vi "Dashboard Main.vi"() -> ()   [LabVIEW 2023]
uses:
  <vilib>/Utility/miscctls.llb/LVRectTypeDef.ctl
  <vilib>/event_ctls.llb/eventvkey.ctl
  <vilib>/Rock Robotics/WPI/DriverStation/WPI_DriverStationAllianceInfo.ctl
  <vilib>/robotics/Kinematics/DH Kinematic Parameters.ctl
  <vilib>/robotics/Kinematics/Link/Joint Type.ctl
  b1c29fd4-b69e-4c47-bd92-218700034153.vi
  cd51690b-7cbe-44fb-a5f0-3232adb0ed53.vi
  a4e8d5d1-2ec3-4e81-be0b-60391cc68073.vi
  1b78be80-bab2-445d-a3e8-82f142a16380.vi
  9e807339-2903-4f51-8fcc-64b6a9381567.vi
  e75f20ac-3dfa-4544-8614-4803d6d17fbb.vi
  273c17a0-a238-4f2a-a55a-7e29d73850ff.vi
  87bdd142-1820-4e26-8582-f713a5f3da40.vi
  b8451b18-7b16-4e07-a196-a1bebf8ce026.vi
  5d307e9f-edd0-4132-a387-09c5916d43b1.vi
  0137daef-9682-45ba-80b9-2d4fda8852b8.vi
  f6a63fab-964b-4051-8314-d4414a0a258c.vi
  90e0fe9d-42b1-4a72-a6c8-4b9d9b3a5a2a.vi
  f15e925d-3118-43e3-bf67-a1272bbf81dd.vi
  394886aa-4cdd-4740-8681-89e3e438764a.vi
  77a42c1f-99bf-4bb6-8218-45b49017f7dc.vi
  5abae45b-ab2b-4816-ba0c-2a0b218f6531.vi
  31f70c1d-3051-4c77-9544-a691198ba614.vi
  f63f5451-5db6-487e-bc86-5cb81e92b132.vi
  81d0db6a-d68a-45c3-b3b1-458879412541.vi
  c235c188-eb56-46fb-93d3-e8acf396af31.vi
  115ba94a-0b26-47fa-ae73-5ec5bd9e502a.vi
  2422668c-951b-48e5-9bda-0f59c56d9c0d.vi
  7776664e-4af7-4b3d-b288-2266642a045e.vi
  321ce103-7778-4bb1-9ecc-75a76fef05e9.vi
  d30e88cc-5e2b-4867-b271-53fc6d5cd4d7.vi
  fde90579-e212-4b8a-8145-a17c3e40bcbd.vi
  6c63589b-432e-4f9c-bacb-2063ed7bd576.vi
  b7dcf304-99f6-4f78-9d14-19aa8d9ea562.vi
  e8b3bb93-ba91-445b-94c6-9e998421f827.vi
  0480a820-69ef-45e6-a9f4-d7ff60c89e45.vi
  1c99237e-ea3d-4ecf-b7c2-61034db3ecd2.vi
  7f172f69-595e-4449-a51b-8be7e20a4729.vi
  02f5d99f-024f-4135-b77d-0032ba8d795b.vi
  0004bdb2-d360-448a-aeac-771fcc1baf3b.vi
  92b8c23e-1d1c-4057-b5e6-223c27eaed30.vi
  7dffb039-adaa-4868-8e10-c58d0581d4f2.vi
  0eb6f919-4c91-4ba7-8f64-447c9ee320a2.vi
  51c227ae-7212-4b29-a489-1f89dd7475d1.vi
  ccddf429-f836-4a79-b987-12239753ca83.vi
  ce254ba4-3e57-42c7-9282-1ab8c635dc3e.vi
  29e0c3c6-4e3c-47cb-b565-5e4554484683.vi
  0a8fe2ab-d060-4915-a9b5-d8978247e2b6.vi
  b1c29fd4-b69e-4c47-bd92-218700034153.vi/77c742ae-e671-49bb-a825-a6e8cebc9f63.vi
  cd51690b-7cbe-44fb-a5f0-3232adb0ed53.vi/77c742ae-e671-49bb-a825-a6e8cebc9f63.vi
  a4e8d5d1-2ec3-4e81-be0b-60391cc68073.vi/77c742ae-e671-49bb-a825-a6e8cebc9f63.vi
  1b78be80-bab2-445d-a3e8-82f142a16380.vi/77c742ae-e671-49bb-a825-a6e8cebc9f63.vi
  9e807339-2903-4f51-8fcc-64b6a9381567.vi/77c742ae-e671-49bb-a825-a6e8cebc9f63.vi
  e75f20ac-3dfa-4544-8614-4803d6d17fbb.vi/77c742ae-e671-49bb-a825-a6e8cebc9f63.vi
  0137daef-9682-45ba-80b9-2d4fda8852b8.vi/77c742ae-e671-49bb-a825-a6e8cebc9f63.vi
  f6a63fab-964b-4051-8314-d4414a0a258c.vi/77c742ae-e671-49bb-a825-a6e8cebc9f63.vi
  90e0fe9d-42b1-4a72-a6c8-4b9d9b3a5a2a.vi/77c742ae-e671-49bb-a825-a6e8cebc9f63.vi
  f15e925d-3118-43e3-bf67-a1272bbf81dd.vi/77c742ae-e671-49bb-a825-a6e8cebc9f63.vi
  394886aa-4cdd-4740-8681-89e3e438764a.vi/77c742ae-e671-49bb-a825-a6e8cebc9f63.vi
  77a42c1f-99bf-4bb6-8218-45b49017f7dc.vi/77c742ae-e671-49bb-a825-a6e8cebc9f63.vi
  5abae45b-ab2b-4816-ba0c-2a0b218f6531.vi/77c742ae-e671-49bb-a825-a6e8cebc9f63.vi
  31f70c1d-3051-4c77-9544-a691198ba614.vi/77c742ae-e671-49bb-a825-a6e8cebc9f63.vi
  f63f5451-5db6-487e-bc86-5cb81e92b132.vi/77c742ae-e671-49bb-a825-a6e8cebc9f63.vi
  81d0db6a-d68a-45c3-b3b1-458879412541.vi/77c742ae-e671-49bb-a825-a6e8cebc9f63.vi
  c235c188-eb56-46fb-93d3-e8acf396af31.vi/77c742ae-e671-49bb-a825-a6e8cebc9f63.vi
  115ba94a-0b26-47fa-ae73-5ec5bd9e502a.vi/77c742ae-e671-49bb-a825-a6e8cebc9f63.vi
  2422668c-951b-48e5-9bda-0f59c56d9c0d.vi/77c742ae-e671-49bb-a825-a6e8cebc9f63.vi
  7776664e-4af7-4b3d-b288-2266642a045e.vi/77c742ae-e671-49bb-a825-a6e8cebc9f63.vi
  321ce103-7778-4bb1-9ecc-75a76fef05e9.vi/77c742ae-e671-49bb-a825-a6e8cebc9f63.vi
  d30e88cc-5e2b-4867-b271-53fc6d5cd4d7.vi/77c742ae-e671-49bb-a825-a6e8cebc9f63.vi
  fde90579-e212-4b8a-8145-a17c3e40bcbd.vi/77c742ae-e671-49bb-a825-a6e8cebc9f63.vi
  6c63589b-432e-4f9c-bacb-2063ed7bd576.vi/77c742ae-e671-49bb-a825-a6e8cebc9f63.vi
  b7dcf304-99f6-4f78-9d14-19aa8d9ea562.vi/77c742ae-e671-49bb-a825-a6e8cebc9f63.vi
  e8b3bb93-ba91-445b-94c6-9e998421f827.vi/77c742ae-e671-49bb-a825-a6e8cebc9f63.vi
  0480a820-69ef-45e6-a9f4-d7ff60c89e45.vi/77c742ae-e671-49bb-a825-a6e8cebc9f63.vi
  1c99237e-ea3d-4ecf-b7c2-61034db3ecd2.vi/77c742ae-e671-49bb-a825-a6e8cebc9f63.vi
  <vilib>/robotics/Kinematics/RotateX.vi
  <vilib>/robotics/Kinematics/RotateY.vi
  <vilib>/robotics/Kinematics/RotateZ.vi
  <vilib>/Analysis/baseanly.llb/A x B.vi
  <vilib>/Analysis/baseanly.llb/Real A x B.vi
  7f172f69-595e-4449-a51b-8be7e20a4729.vi/77c742ae-e671-49bb-a825-a6e8cebc9f63.vi
  02f5d99f-024f-4135-b77d-0032ba8d795b.vi/77c742ae-e671-49bb-a825-a6e8cebc9f63.vi
  0004bdb2-d360-448a-aeac-771fcc1baf3b.vi/77c742ae-e671-49bb-a825-a6e8cebc9f63.vi
  92b8c23e-1d1c-4057-b5e6-223c27eaed30.vi/77c742ae-e671-49bb-a825-a6e8cebc9f63.vi
  7dffb039-adaa-4868-8e10-c58d0581d4f2.vi/77c742ae-e671-49bb-a825-a6e8cebc9f63.vi
  29e0c3c6-4e3c-47cb-b565-5e4554484683.vi/77c742ae-e671-49bb-a825-a6e8cebc9f63.vi
  0a8fe2ab-d060-4915-a9b5-d8978247e2b6.vi/77c742ae-e671-49bb-a825-a6e8cebc9f63.vi
  <vilib>/Rock Robotics/Network Tables/NT Read Number.vi
  <vilib>/Rock Robotics/Network Tables/NT Read Boolean.vi
  GlobalDashboard.vi
  <vilib>/Rock Robotics/Network Tables/NT Read String.vi
  <vilib>/Rock Robotics/Network Tables/NT Write Number.vi
  <vilib>/Rock Robotics/Network Tables/NT Read Numeric Array.vi
  <vilib>/Rock Robotics/Network Tables/NT Read String Array.vi
  <vilib>/Rock Robotics/Network Tables/NT Write Boolean.vi
  <vilib>/Rock Robotics/Network Tables/NT Read Boolean Array.vi
  <vilib>/Rock Robotics/Network Tables/NT Write String.vi
  <vilib>/Rock Robotics/Network Tables/NT Write Numeric Array.vi
  <vilib>/picture/3D Picture Control/Object/Add Object (no reference).vi
  <vilib>/Rock Robotics/Network Tables/NT Write String Array.vi
  <vilib>/Utility/xml.llb/Write to XML File(string).vi
  <vilib>/Utility/xml.llb/Read From XML File(array).vi
  <vilib>/picture/3D Picture Control/Object/Create Object (drawable).vi
  <vilib>/Rock Robotics/Network Tables/NT Read Integer.vi
  <vilib>/robotics/Kinematics/Analytical/Initialize Generic Serial Arm.vi
  <vilib>/vision/NI_Vision_Development_Module.lvlib
  <vilib>/robotics/Kinematics/Link/NI_Robotics_Link.lvclass
  <vilib>/robotics/Kinematics/Analytical/NI_Robotics_AnalyticKinematics.lvlib
  <vilib>/robotics/Kinematics/Robot/NI_Robotics_Serial Robot Arm.lvclass
  <vilib>/robotics/Kinematics/NI_Kinematics.lvlib
  <vilib>/picture/3D Picture Control/NI_3D Picture Control.lvlib
  <vilib>/robotics/Kinematics/Plotting/NI_Robotics_3DKinematics.lvlib
panel:
  out "Shooter_Fault_Array":bool[](array[boolean])
  out "Shooter_Overheating_Array":bool[](array[boolean])
  in  "TCP":refnum<k5>
  in  "Dashboard Tab":T1(tab)=enum."Setup/Auto"
  in  "CheckList":i32(listbox)
  in  "Launch_Camera":bool
  out "Distance_to_Target":dbl format="%.1f"
  in  "Enable_Streaming_GUI":bool=TRUE
  out "Robot_Profile_GUI":string
  out "Auto_Playbook_GUI":string
  in  "Select Driver Profile":u16(ring) items=["N/A"]
  in  "Camera Name":string(combo)="limelight"
  in  "Camera Settings":T2={"Frame Rate"=20, "Compression"=60, "Size"=1, "DB Camera Config"=FALSE} {"Size" items=["640x480", "320x240", "160x120"]}
  in  "Select Autonomous Play":u16(ring) items=["N/A"]
  out "Master_Caution_GUI_0":bool caption="Mode_Butterfly"
  out "Robot_is_Autonomous_GUI_0":bool caption="Mode_Butterfly"
  out "Robot_Code_Version_GUI":string
  out "Auto_Suffix_GUI":string
  in  "Refresh_Auto_Play_List_GUI":bool
  in  "Auto_Delay_GUI":dbl format="%.1f"
  in  "Manual_Start_X":dbl min=0.0 max=700.0 format="%.1f"
  out "Robot_X":dbl format="%.1f"
  out "Robot_Y":dbl format="%.1f"
  in  "Manual_Start_Y":dbl min=0.0 max=400.0 format="%.1f"
  out "Robot_H_GUI":dbl format="%.1f"
  in  "Manual_Start_H":dbl min=0.0 max=360.0 format="%.1f"
  in  "Field Map":u16(ring) items=["N/A"]
  in  "Push_Robot_Start_GUI":bool
  in  "Export_Robot_Pose":bool
  in  "Clear_Robot_Pose_Display":bool
  in  "Dock_Dashboard":bool
  in  "Force_Human_Control_GUI":bool
  in  "Auto_Test_Mode_GUI":bool
  in  "Disable_Fusion_While_Autonomous":bool
  in  "Disable_Fusion_While_Disabled":bool=TRUE
  out "Robot Pose 1":cluster{dbl[], dbl[]}[](graph)
  in  "Camera Switch\nCamera Switch":bool
  out "Master_State_STOW_Indicator":bool
  in  "Elevator_Override":bool
  in  "Wrist_Override":bool
  out "(Front) Lemon_Vision_Fault_GUI":bool
  out "Shooter_State_STGE":bool
  out "Shooter_State_SUBW":bool
  out "Shooter_State_TACO":bool
  out "Note 2":bool caption="Mode_Butterfly"
  out "Wrist_Motor_Fault":bool
  out "Wrist_Overheating":bool
  out "Ready_To_Fire":bool caption="Mode_Butterfly"
  out "Shooter_Right_Overheating":bool
  out "Shooter_Motor_Right_Fault":bool
  out "Outtaking":bool caption="Mode_Butterfly"
  out "Intaking":bool caption="Mode_Butterfly"
  out "Shooter_Motor_Left_Fault":bool
  out "Shooter_Left_Overheating":bool
  out "Indexer_Overheating":bool
  out "Indexer_Motor_Fault":bool
  out "Intake_Motor_Fault":bool
  out "Intake_Overheating":bool
  out "Elevator_Motor_Fault":bool
  out "Elevator_Overheating":bool
  out "Master_State_TRAP_Indicator":bool
  out "Master_State_CLIMB_Indicator":bool
  out "Master_State_AMP_Indicator":bool
  out "Help Graphic":T3(plugin-control)
  out "LL_Ret_Left":bool
  out "LL_Ret_Right":bool
  out "WA_Ret_Right":bool
  out "WA_Ret_Left":bool
  out "Swerve_Drive_Fault":bool
  out "Robot Pose 2":cluster{dbl[], dbl[]}[](graph)
  out "Master_State_SPEAKER_Indicator":bool
  out "(Back) Lime_Vision_Fault_GUI":bool
  out "Pressure_Leak_GUI":bool
  in  "Master_Safety_Override_1":bool
  in  "Manipulator_Help":bool
  in  "Driver_Help":bool
  out "No_Secondary_Camera":bool
  out "Electrical_Fault_GUI":bool
  out "Diverting_Power_GUI":bool
  out "CAN_Bus_Fault_GUI":bool
  out "IMU_Failure_GUI":bool
  out "Robot_is_Autonomous_GUI_1":bool caption="Mode_Butterfly"
  out "LL_Valid":bool caption="Mode_Butterfly"
  out "Auto_Error_GUI":bool
  in  "Clear_Errors_GUI":bool
  out "Swerve_Azimuth_Fault":bool
  out "Pressure_Transducer_GUI":dbl(slide) scale=0.0..115.0
  out "Pressure_Vent_GUI":bool
  out "Swerve_Overheating":bool
  out "Compressor_On_GUI":bool
  in  "Right":bool
  in  "Reticule":T4(ring)
  in  "Save":bool
  in  "Up":bool
  in  "Down":bool
  in  "Left":bool
  out "Master_Caution_GUI_1":bool caption="Mode_Butterfly"
  out "Battery_Critical_GUI":bool
  out "Battery_Voltage_GUI":dbl(slide) scale=11.0..13.0
  out "Field_Oriented_GUI":bool caption="Mode_Butterfly"
  out "Slow_Loop":bool
  out "Combined Camera Feed":T3(plugin-control)
  in  "Field_Oriented_Override_GUI":bool
  in  "Auto_Targeting_Override":bool
  out "Using_Auto_Targeting":bool caption="Mode_Butterfly"
  out "Elevator_Has_Arrived":bool caption="Mode_Butterfly"
  out "Pivot_Position (deg)":dbl format="%.1f"
  out "Pivot_Temp (C)":dbl
  in  "Unlock_Pivot":bool
  out "Wrist_Position (deg) 2":dbl format="%.1f"
  out "Wrist_Temp (C) 2":dbl
  in  "Unlock_Wrist":bool
  out "Swerve_Output_Loop_Time_GU":u32
  out "Swerve_3_Drive_Velocity":dbl format="%.1f"
  out "Swerve_3_Azimuth_Position":dbl format="%.1f"
  out "Swerve_3_Drive_Temperature":dbl
  out "Swerve_0_Drive_Temperature":dbl
  out "Camera Perf":string
  out "Control_Loop_Time_GUI":u32
  in  "Calibrate_Wheels_GUI":bool
  in  "Home_Wheels_GUI":bool
  out "Swerve_0_Azimuth_Position":dbl format="%.1f"
  out "Swerve_0_Drive_Velocity":dbl format="%.1f"
  out "Swerve_1_Drive_Velocity":dbl format="%.1f"
  out "Swerve_1_Azimuth_Position":dbl format="%.1f"
  out "Swerve_1_Drive_Temperature":dbl
  out "Swerve_2_Drive_Velocity":dbl format="%.1f"
  out "Swerve_2_Azimuth_Position":dbl format="%.1f"
  out "Swerve_2_Drive_Temperature":dbl
  in  "Arm_Calibrate_Wheels_GUI":bool
  out "Master_Caution_GUI_2":bool caption="Mode_Butterfly"
  in  "Actuator Testing":u16(ring) items=["N/A"]
  in  "Test_Actuator_Value_GUI":dbl step=0.1 format="%.2f"
  in  "Calibrate_Joysticks_GUI":bool
  in  "Arm_Calibrate_Joysticks":bool
  out "Robot_is_Autonomous_GUI_2":bool caption="Mode_Butterfly"
  in  "Test_Actuator_Period_GUI":dbl min=0.0 step=1.0 format="%.2f"
  out "Pose_Loop_Time_GUI":u32
  in  "Mute_Audible_Warnings":bool
  out "Combined Error String":string
  out "Swerve_0_Shifter_State":string
  out "Swerve_1_Shifter_State":string
  out "Swerve_3_Shifter_State":string
  out "Swerve_2_Shifter_State":string
  out "Swerve_Azimuth_Fault_Array":bool[](array[boolean])
  in  "Super_Test_Mode_GUI":bool
  out "Current_Driver_Profile_Setpoints_GUI":T5={"Strafe Deadband"=0.08, "Strafe Scaling"=2.0, "Strafe Maximum"=0.5, "Rotation Deadband"=0.15, "Rotation Scaling"=2.5, "Rotation Maximum"=0.5} {"Rotation Maximum" min=0.3 max=1.0 scale=0.3..1.0; "Rotation Scaling" min=1.0 max=4.0 scale=1.0..4.0; "Rotation Deadband" min=0.0 max=0.25 scale=0.0..0.25; "Strafe Maximum" min=0.3 max=1.0 scale=0.3..1.0; "Strafe Scaling" min=1.0 max=4.0 scale=1.0..4.0; "Strafe Deadband" min=0.0 max=0.25 scale=0.0..0.25}
  in  "New_Driver_Profile_Setpoints_GUI":T6={"Strafe Deadband"=0.08, "Strafe Scaling"=2.0, "Strafe Max"=0.5, "Rotate Deadband"=0.15, "Rotate Scaling"=2.5, "Rotate Max"=0.5} {"Rotate Max" min=0.3 max=1.0 format="%.2g"; "Rotate Scaling" min=1.0 max=4.0 format="%.2g"; "Rotate Deadband" min=0.0 max=0.25 format="%.2g"; "Strafe Max" min=0.3 max=1.0 format="%.2g"; "Strafe Scaling" min=1.0 max=4.0 format="%.2g"; "Strafe Deadband" min=0.0 max=0.25 format="%.2g"}
  in  "Apply_Driver_Profile_Setpoints_GUI":bool
  out "Current_Driver_Profile_GUI":string
  in  "Free_Tuning_Variable_GUI":dbl min=0.0 step=1.0 format="%.3f"
  out "Audible_Warnings_Enabled_GUI":bool
  out "Legal_Drivers_GUI":string[](array[string])
  out "Swerve_Overheating_Array":bool[](array[boolean])
  out "Swerve_Drive_Fault_Array":bool[](array[boolean])
  out "Intake_Motor_Fault_Array":bool[](array[boolean])
  out "Intake_Overheating_Array":bool[](array[boolean])
  out "Extender_Position (deg)":dbl format="%.1f"
  out "Extender_Temp (C)":dbl
  in  "Calibrate_Extender":bool
  in  "Unlock_Extender":bool
  out "State_AMP":bool
  out "State_Climbing":bool
  out "NT Connection":bool
  out "Mode":T7(ring)=enum."Auto Disabled"
  out "Tree":string(tree)
  out "Background":bool
  # "2025 Dashboard v1.0-dev"
  # "Robot Profile"
  # "Robot X Position (in)"
  # "Robot Y Position (in)"
  # "Delay (s)"
  # "Robot Heading (deg)"
  # "Suffix"
  # "X (in)"
  # "Robot Pitch (deg)"
  # "Autonomous Playbook Entry"
  # "Auto Test\nMode"
  # "Force\nHuman"
  # "Y (in)"
  # "Target Distance (in)"
  # "H (deg)"
  # "Undock Dashboard"
  # "Yes Camera Streaming"
  # "Stop Fusion While Auto"
  # "Stop Fusion While Disabled"
  # "X"
  # "Y"
  # "MASTER\nSTATES"
  # "OVERRIDES"
  # "Robot-Oriented Drive Controls"
  # "Camera Switch"
  # "Auto-Targeting Override"
  # "Wrist\nOverride"
  # "SHOOTER\nSTATES"
  # "Arm\nOverride"
  # "Disengage\nSafeties"
  # "11"
  # "13"
  # "0"
  # "120"
  # "Drivebase Subsytem"
  # "Driver Profile Selected"
  # "Loop Times"
  # "Module 1"
  # "Module 0"
  # "Control (ms)"
  # "Azimuth (deg)"
  # "Pose (ms)"
  # "Temp (C)"
  # "Drive Output (ms)"
  # "Velocity (ft/s)"
  # "Shifter State"
  # "Module 2"
  # "Module 3"
  # "Variable (bleh)"
  # "Disabled\nTest Mode"
  # "Azimuth (deg)"
  # "Temp (C)"
  # "Velocity (ft/s)"
  # "Arm Subsystem"
  # "Shifter State"
  # "Calibrate Extender"
  # "Unlock Wrist"
  # "Unlock Pivot"
  # "Calibrate Wheels"
  # "Gripper Subsystem"
  # "Extender"
  # "Extender"
  # "Extender"
  # "Period (s)"
  # "Calibrate Joysticks"
  # "Amplitude"
  # "Velocity (rpm)"
  # "Position (in)"
  # "Pos (deg)"
  # "Pos (deg)"
  # "Temp (C)"
  # "Temp (C)"
  # "Temp (C)"
  # "Temp (C)"
  # "0"
  # "0.25"
  # "1"
  # "4"
  # "0.3"
  # "1"
  # "0"
  # "0.25"
  # "1"
  # "4"
  # "0.3"
  # "1"
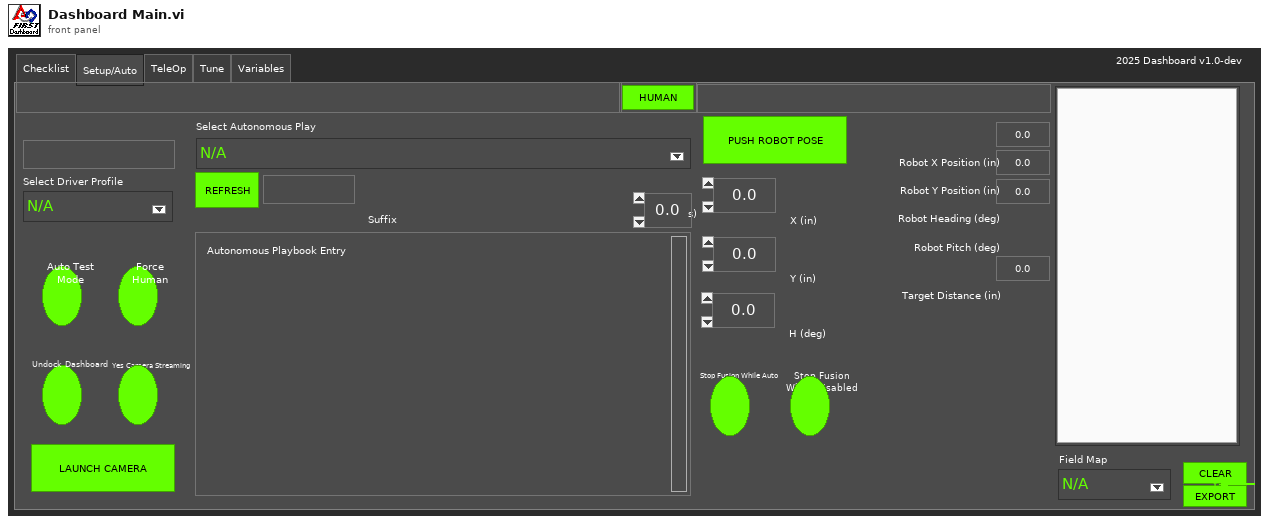
[diagram p1: front panel]
types:
  T1 = enum32{"Checklist", "Setup/Auto", "TeleOp", "Tune", "NT", "Test", "Commands", "Variables"}
  T2 = cluster{"Frame Rate":i32, "Compression":i32, "Size":u16, "DB Camera Config":bool}
  T3 = typedef "IMAQ Image.ctl" = refnum<image>
  T4 = enum16{"Wide Angle Left Reticule", "Wide Angle Right Reticule", "Lime Light Left Reticule", "Lime Light Right Reticule"}
  T5 = cluster{"Strafe Deadband":dbl, "Strafe Scaling":dbl, "Strafe Maximum":dbl, "Rotation Deadband":dbl, "Rotation Scaling":dbl, "Rotation Maximum":dbl}
  T6 = cluster{"Strafe Deadband":dbl, "Strafe Scaling":dbl, "Strafe Max":dbl, "Rotate Deadband":dbl, "Rotate Scaling":dbl, "Rotate Max":dbl}
  T7 = enum8{"Tele-Op Disabled", "Tele-Op Enabled", "Auto Disabled", "Auto Enabled", "Test Disabled", "Test Enabled", "Disconnected", "No Code", "E-Stop"}
  T8 = cluster{"Save Path":path, "Interval (s)":dbl, "Keep":i32}
  T9 = enum32{"Drive", "Camera", "Basic", "Custom", "Test", "Commands", "Checklist", "Variables"}
  T10 = cluster{"IDs":cluster{"RPC field ID":u16, "Unique ID":u16}, "String":string}
  T11 = typedef "Image Type" = u32
  T12 = cluster{"Camera Name":string, string, "Saved DB Images Info":cluster{"Save Path":path, "Interval (s)":dbl, "Keep":i32}}
  T13 = typedef "WPI_DriverStationAllianceInfo.ctl" = enum16{"Red", "Blue", "Invalid"}
  T14 = cluster{"Red":sgl, "Green":sgl, "Blue":sgl, "Alpha":sgl}
  T15 = typedef "DH Kinematic Parameters.ctl" = cluster{"twist angle":dbl, "length":dbl, "rotation angle":dbl, "offset distance":dbl, "joint type":T16, "joint coordinate offset":dbl}
  T16 = typedef "NI_Robotics_Link.lvclass/Joint Type.ctl" = enum16{"Revolute", "Prismatic"}
  T17 = enum8{"Enabled", "Disabled", "Disabled and Grayed Out"}
  T18 = cluster{"Error Strings":string, "Disable Counts":cluster{u16, u16}, "Rail Faults":cluster{u16, u16, u16}, "Robot IP":string, "DB Mode":u8, "Event Info":cluster{"Name":string, "Type":u8, "Number":u16, "Replay":u8}}
  T19 = cluster{"Storage":cluster{"Disk Free":u64, "RAM Block":u32, "RAM free":u32}, "CPU Utilization":cluster{"CPU % ISR":sgl, "CPU % Time Crit":sgl, "CPU % Timed Str":sgl, "CPU % High":sgl, "CPU % Above":sgl, "CPU % Normal":sgl, "CPU % Low":sgl}, "CAN":cluster{"% Bus Utilization":sgl, "Bus Off Cnt":u32, "TX_FIFO Full Cnt":u32, "Receive Error Cnt":u8, "Transmit Error Cnt":u8}, "HID":cluster{"HID Outputs":u32, "Rumble Low":u16, "Rumble High":u16}[]}
  T20 = cluster{"Status bits":cluster{"Test Mode":bool, "Autonomous":bool, "Enabled":bool, "Code Start":bool, "Brownout":bool, "Reserved 2":bool, "Reserved 3":bool, "E-Stop":bool}, "Code Trace":cluster{"Disabled":bool, "TeleOp":bool, "Auto":bool, "Test":bool}, "Controller Type":enum16{"unknown", "cRIO", "roboRio"}, "Code?":enum16{"unknown", "noCode", "code"}, "Battery V":dbl}
  T21 = cluster{"Control Bits":cluster{"TestMode":bool, "Autonomous":bool, "Enabled":bool, "FMS Present":bool, bool, bool, bool, "E-Stop":bool}, "Team Station ":u8, "Countdown":sgl, "Joystick Values":cluster{"Axes":dbl[], "Buttons":bool[], "POVs":i16[]}[]}
  T22 = typedef "imagedata.ctl" = cluster{"image type":i32, "image depth":i32, "image":u8[], "mask":u8[], "colors":u32[], "Rectangle":cluster{"left":i16, "top":i16, "right":i16, "bottom":i16}}
  T23 = cluster{"Boolean":bool, "Numeric Text.Text Colors:Text Color":u32}
  T24 = cluster{"value[0]":dbl, "value[1]":dbl, "value[2]":dbl, "value[3]":dbl, "value[4]":dbl, "value[5]":dbl}
  T25 = typedef "NI_Matrix.lvlib/RealMatrix.ctl" = dbl[][]
  T26 = typedef "LVRectTypeDef.ctl" = cluster{"Left":i16, "Top":i16, "Right":i16, "Bottom":i16}
  T27 = typedef "eventvkey.ctl" = enum16{"ASCII", "Enter", "Return", "Shift", "Ctrl", "Alt", "Cmd", "Opt", "Caps", "NumLock", "Clear", "Break", "Up", "Down", "Left", "Right", "Insert", "Delete", "Home", "End", "PageUp", "PageDown", "Escape", "Help", "Pause", "ScrollLock", "F1", "F2", "F3", "F4", "F5", "F6", "F7", "F8", "F9", "F10", "F11", "F12", "F13", "F14", "F15", "F16", "F17", "F18", "F19", "F20", "F21", "F22", "F23", "F24", "Play", "VolumeUp", "VolumeDown", "Mute", "Two Byte Char"}
  T28 = cluster{"Shift":bool, "Ctrl":bool, "Alt":bool, "Cmd":bool, "Opt":bool}
  T29 = cluster{"WA_Ret_Left":refnum<vi>, "WA_Ret_Right":refnum<vi>, "LL_Ret_Left":refnum<vi>, "LL_Ret_Right":refnum<vi>}
  T30 = cluster{string, "(Back) Lime_Vision_Fault_GUI":bool, dbl}
  T31 = cluster{string, "Elevator_Motor_Fault":bool, dbl}
  T32 = cluster{string, "Elevator_Overheating":bool, dbl}
  T33 = cluster{string, "Master_Safety_Override_1":bool, dbl}
  T34 = cluster{string, "Swerve_Azimuth_Fault":bool, dbl}
  T35 = cluster{string, "Arm_Calibrate_Wheels_GUI":bool, dbl}
  T36 = cluster{string, "Electrical_Fault_GUI":bool, dbl}
  T37 = cluster{string, "Arm_Calibrate_Joysticks":bool, dbl}
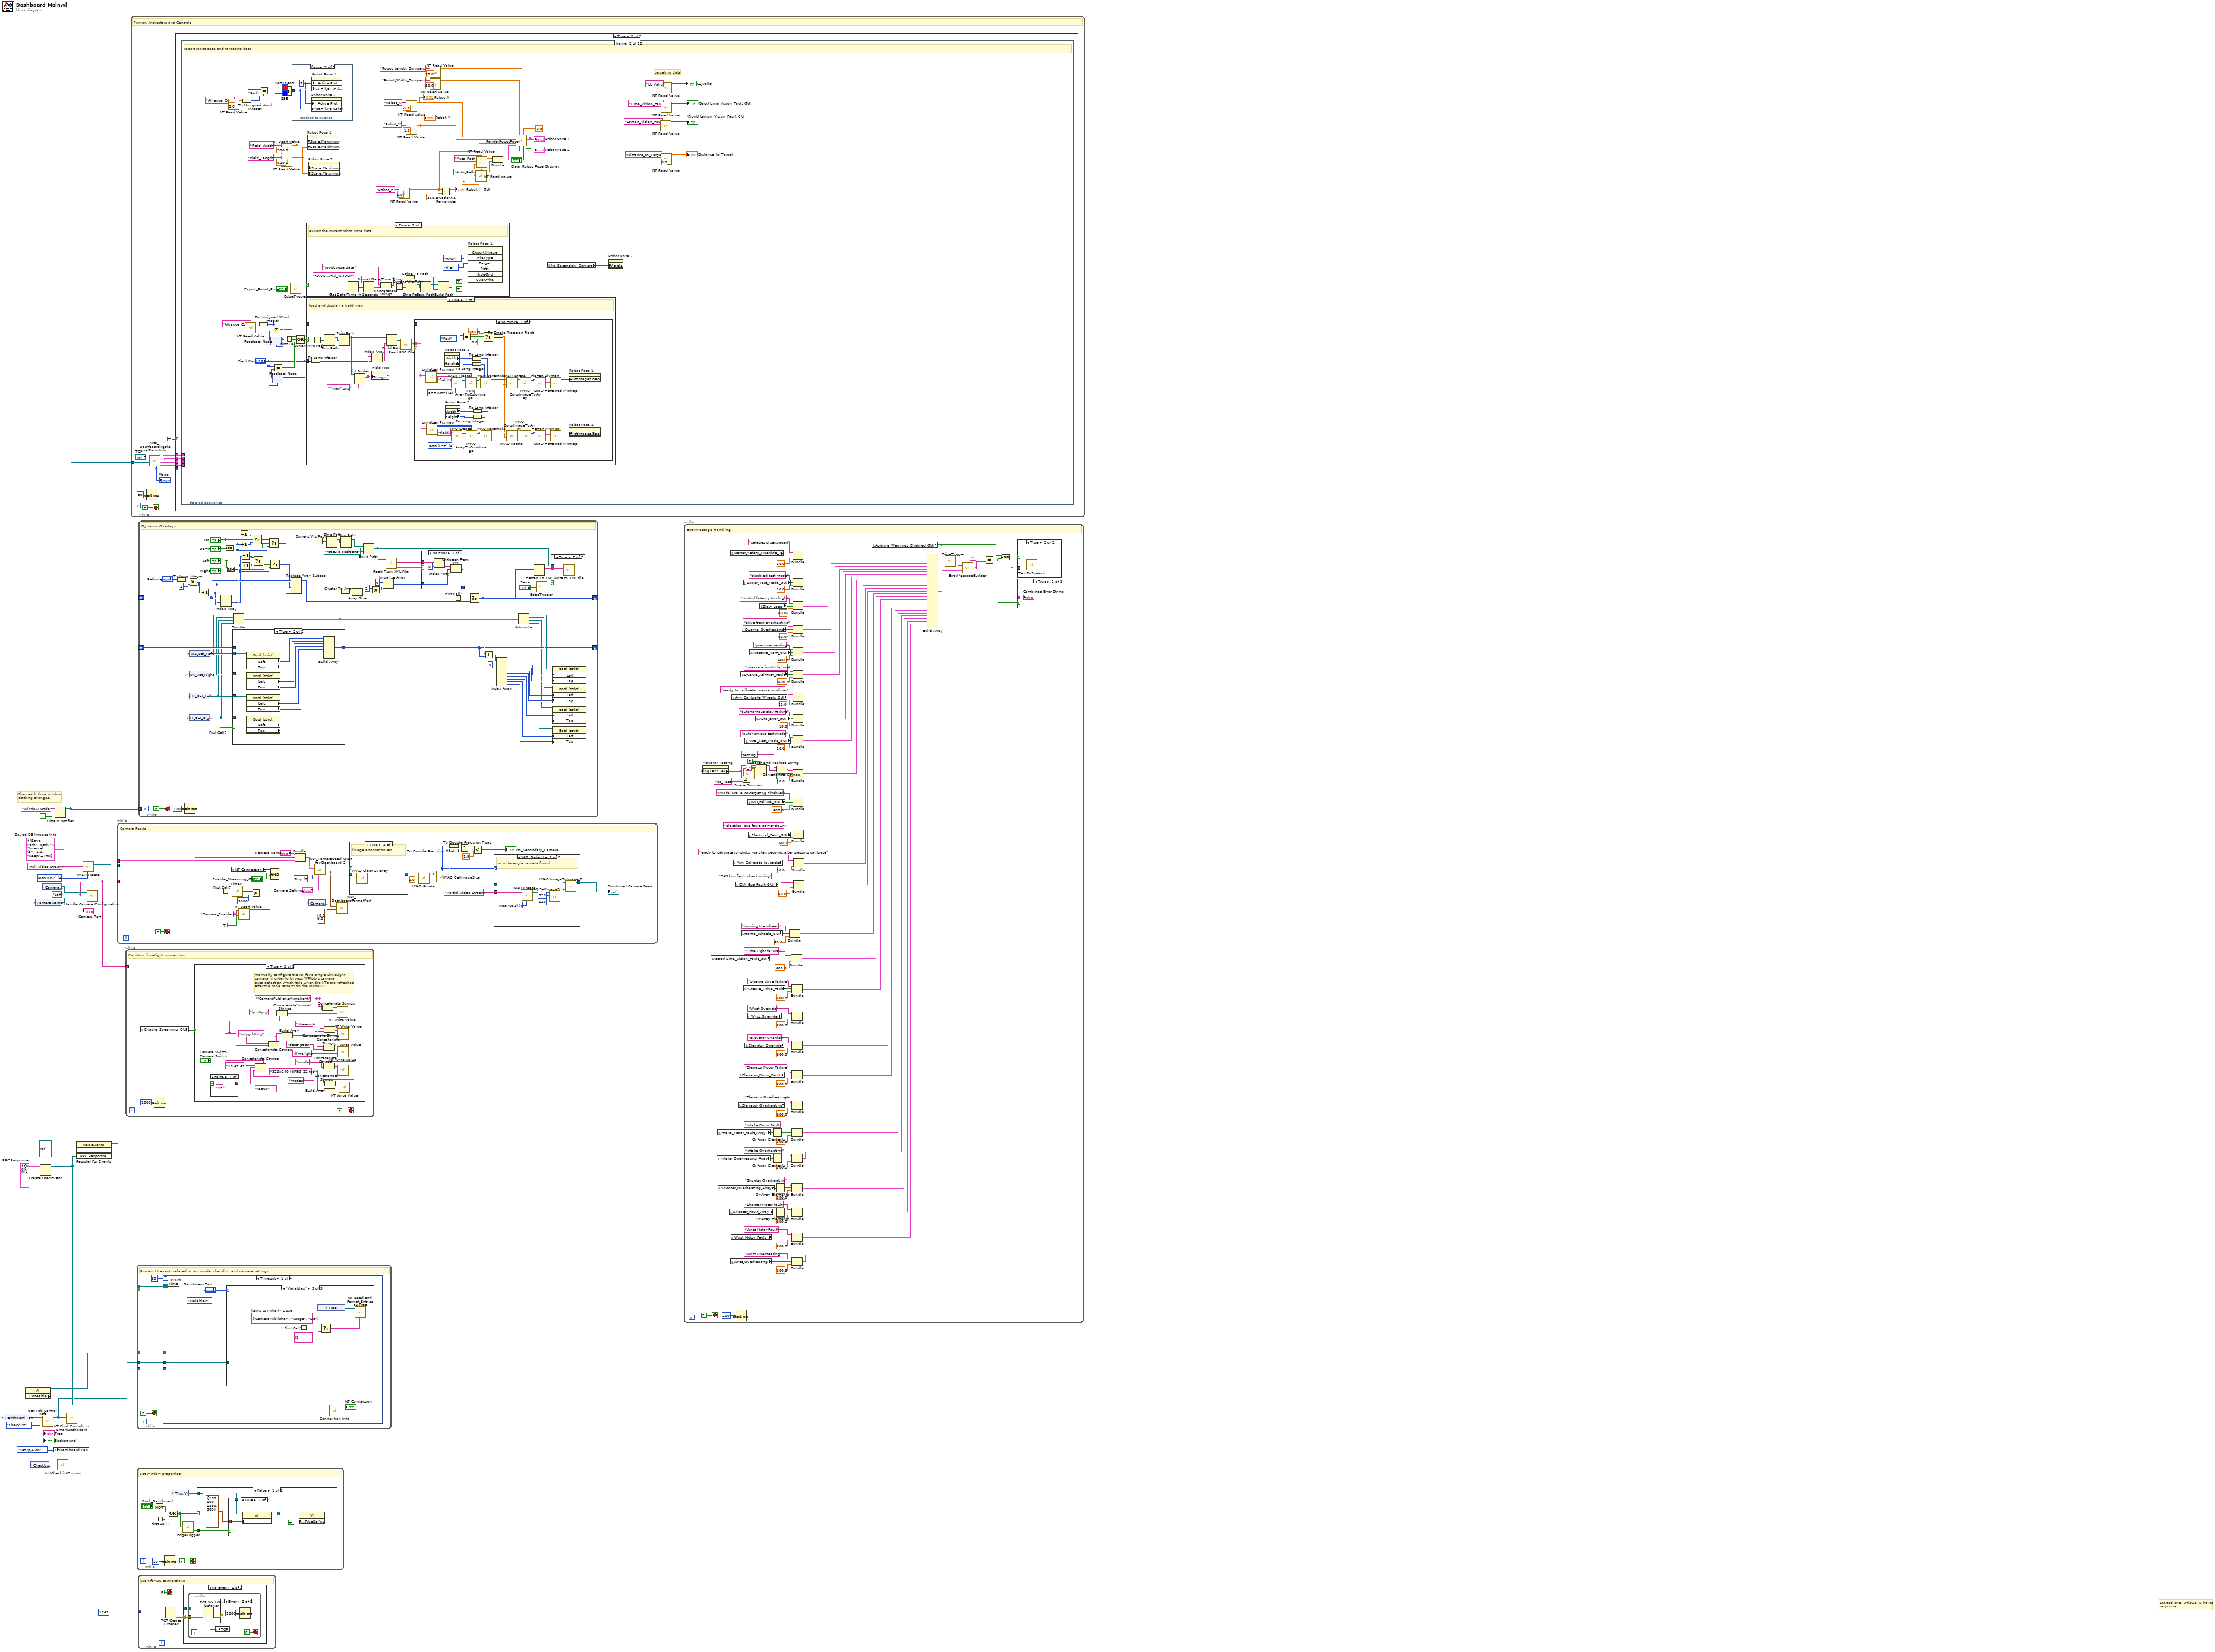
[diagram p0: block diagram]
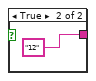
[diagram p3: hidden frame]
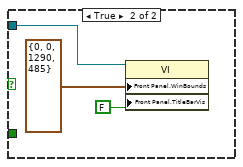
[diagram p5: hidden frame]
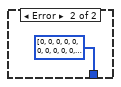
[diagram p8: hidden frame]
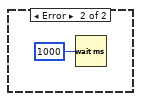
[diagram p12: hidden frame]
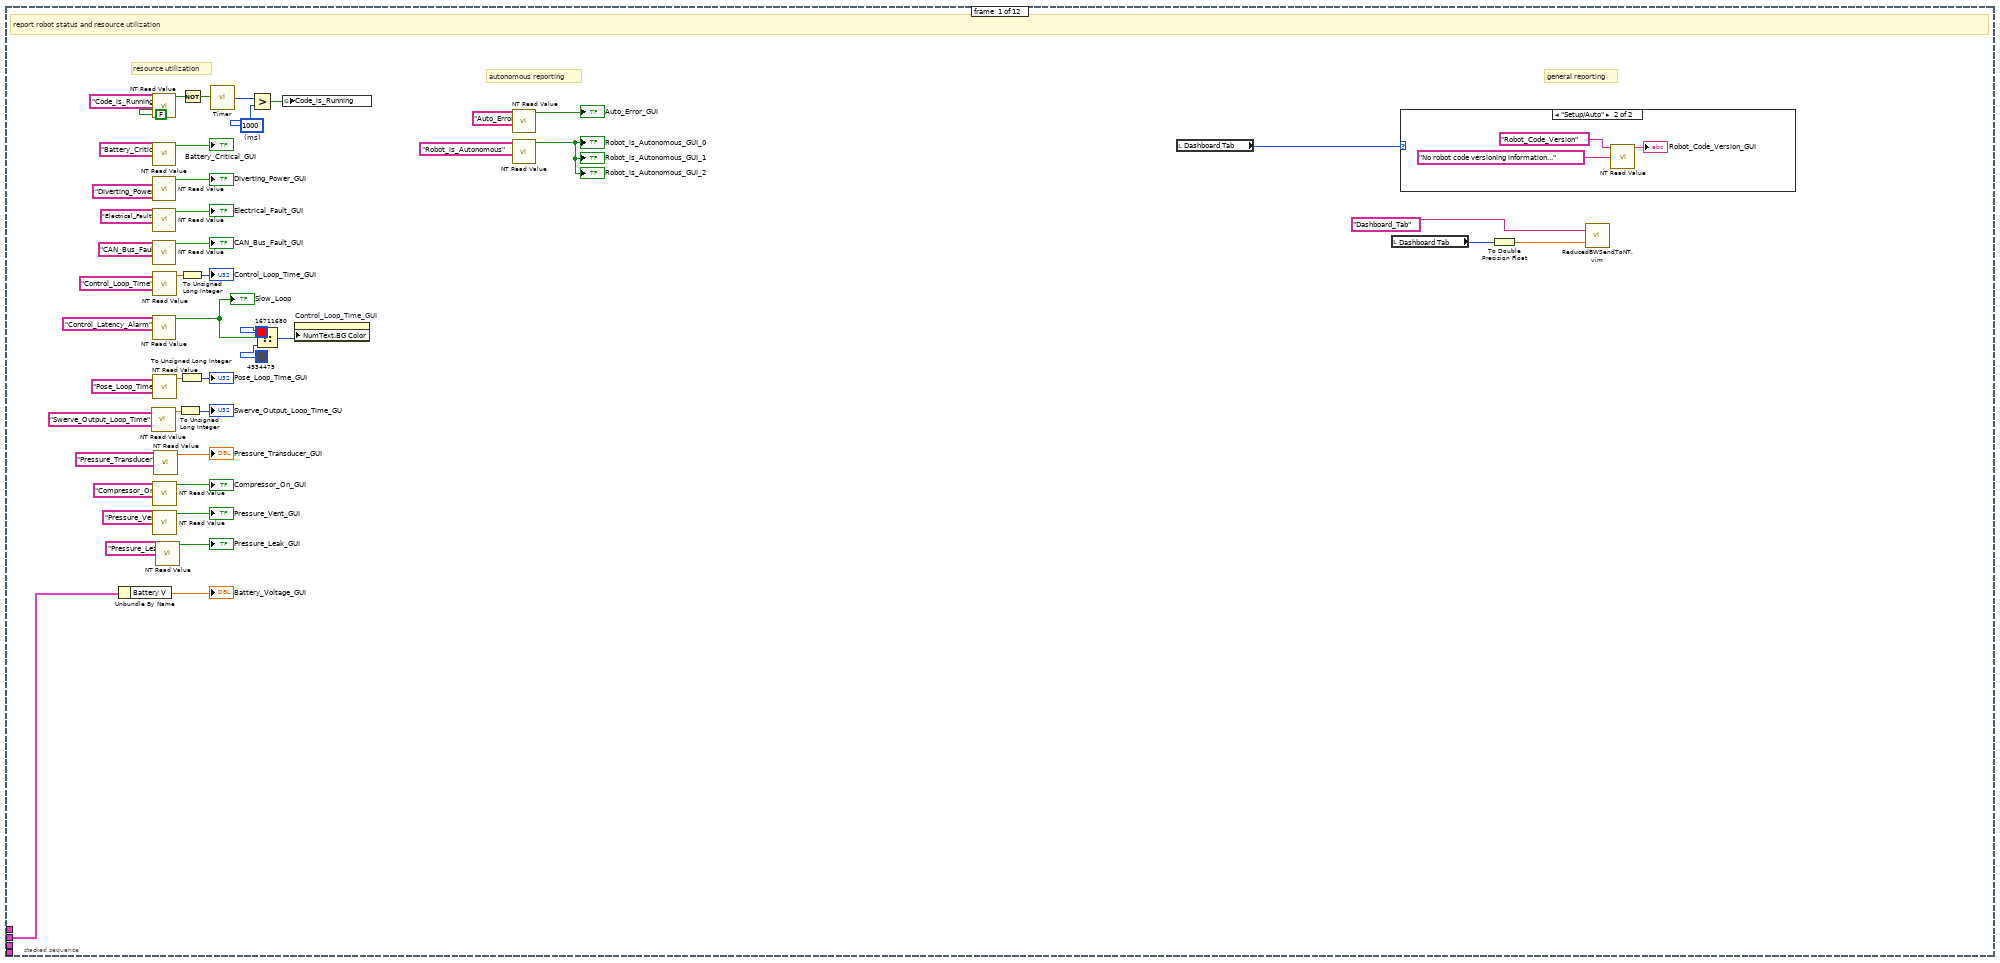
[diagram p14: hidden frame]
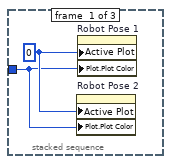
[diagram p16: hidden frame]
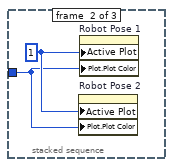
[diagram p17: hidden frame]
diagram:
  w10 = T8 {"Save Path"=path "", "Interval (s)"=1.0, "Keep"=180}  # Saved DB Images Info
  w2 = "Left"
  w13 = T10 {"IDs"={"RPC field ID"=0, "Unique ID"=0}, "String"=""}  # RPC Response
  w8 = T11 4 items=["Grayscale (U8)", "Grayscale (I16)", "Grayscale (SGL)", "Complex (CSG)", "RGB (U32)", "HSL (U32)", "RGB (U64)"] ("Image Type")
  # "Started one, Unique ID holds\nresponse"
  # "Fires each time window\ndocking changes."
  n1 = control-ref of="Dashboard Tab"() -> (w16:refnum<vi>)
  n2 = property class="VI" props=["Front Panel.Closeable"]() -> (reference out=w17:refnum<vi>)  [unwired: 2 in, 2 out]
  n3 = control-ref of="CheckList"() -> (w7:refnum<vi>)
  n4 = control-ref of="Camera Name"() -> (w1:refnum<vi>)
  n5 = Create User Event(user event datatype=w13) -> (user event=w12:refnum<user-event>)  [unwired: 1 in, 1 out]
  n6 = control-ref of="Camera Settings"() -> (w3:refnum<vi>)
  n7 = call <vilib>:"Get Tab Control Refs.vi"("Page Index"=T9."Checklist" ("Dashboard Tab"), "TabControl in"=w16) -> ("ControlsOnPage"=w5:refnum<vi>[])  [unwired: 9 in]
  n8 = local write "Dashboard Tab"(T1."Setup/Auto" ("Dashboard Tab")) -> ()
  n9 = Obtain Notifier(name (unnamed)="Window Mode", notification data type=TRUE) -> (notifier out=w4:refnum<notifier>)  [unwired: 2 in, 2 out]
  n10 = call "InitChecklistCustom.vi"("ListBox in"=w7) -> ()  [unwired: 1 in]
  n11 = call <vilib>:"NT Bind Controls to SmartDashboard.vi"("Bound Control Refs"=w5) -> ()  [unwired: 11 in]
  n12 = register-events(refnum<vi> refnum, w12) -> (reference out=w20:refnum<event-registration>, error out=w19:errorcluster)  [unwired: 2 in]
  n13 = call "IMAQ Create"("Image Name"="Full Video Stream", "Image Type"=w8) -> ("New Image"=w6:T3)  [unwired: 2 in, 2 out]
  n14 = call "Handle Camera Configuration.vi"("CameraNameRef"=w1, "Display Name"=w2, "ClusterRef"=w3) -> ()  [unwired: 9 in]
  n15 = while {
    tunnel: w10 -> [w56]
    tunnel: w2 -> [w55]
    tunnel: w6 -> [w54]
    stop <- FALSE stop-if-true
    w26 = u16 0 items=["Stop", "Record", "Playback Panel"] ("Rec Mode")
    # "Camera Feeds"
    n16 = First Call?() -> (First Call?: T/F=w33:bool)
    n17 = local read "NT Connection"() -> (w36:bool)
    n18 = call "Timer.vi"("Reset Timer"=w33) -> ("Time (ms)"=w32:u32)
    n19 = call-poly <vilib>:"NT Read Value.vi"("default value"=TRUE, "name"="Camera_Enabled") -> ("value"=w24:bool)  [unwired: 7 in, 2 out]
    n20 = Greater?(x=w32, y=u32 5000) -> (0:w30:bool)
    n21 = Compound Arithmetic op=AND(w36, "Enable_Streaming_GUI", w30, w24) -> (w35:bool)
    n22 = Bundle("Camera Name"="Camera Name", w55, "Saved DB Images Info"=w56) -> (w52:T12)  [unwired: 1 in]
    n23 = control-ref of="Camera Perf"() -> (w50:refnum<vi>)
    n24 = call <vilib>:"WPI_CameraRead MJPG for Dashboard_2.vi"("Camera Settings"="Camera Settings", "Rec Mode"=w26, "NT Connection"=w35, "Capture Info"=w52, "Image in"=w54) -> ("perf info"=w51:cluster{"Bandwidth (Mbps)":dbl, "fps":dbl}, "Active"=w37:bool, "Image\\ out"=w53:T3)  [unwired: 4 in]
    n25 = call <vilib>:"WPI_DashboardFormatPerf.vi"("Right Camera Perf"=cluster{"Bandwidth (Mbps)":dbl, "FPS":dbl} {"Bandwidth (Mbps)"=0.0, "FPS"=0.0}, "Performance"=w51, "String in"=w50) -> ()  [unwired: 9 in]
    n26 = case shown="True" w37 {
      tunnel: w53 -> [w67 w70]
      tunnel: [w67 w69] -> w49
      frame False {
        n27 = Wait Until Next ms Multiple(millisecond multiple=u32 500) -> ()  [unwired: 1 out]
      }
      frame True {
        # "image annotation etc."
        n28 = call "IMAQ Clear Overlay"("Image"=w70) -> ("Image Out"=w69:T3)  [unwired: 2 in, 8 out]
      }
    }
    n29 = call "IMAQ Rotate"("Angle (degrees)"=sgl 0.0, "Image Src"=w49) -> ("Image Dst Out"=w40:T3)  [unwired: 8 in, 1 out]
    n30 = call "IMAQ GetImageSize"("Image"=w40) -> ("Y Resolution"=w38:i32, "X Resolution"=w27:i32)  [unwired: 3 in, 1 out]
    n31 = To Double Precision Float(number=w27) -> (double precision float=w47:dbl)
    n32 = To Double Precision Float(number=w38) -> (double precision float=w46:dbl)
    n33 = Divide(x=w47, y=w46) -> (x/y=w45:dbl)
    n34 = Less?(x=w45, y=1.9) -> (x < y?=→"No_Secondary_Camera":bool)
    n35 = case shown="160, Default" w27 {
      tunnel: "Partial Video Stream" ("Image Name") -> [_ w66]
      tunnel: [w58 w65] -> w29
      tunnel: w40 -> [w58 w63]
      frame 320 {
        # "wide angle camera found"
      }
      frame 160, Default {
        w59 = T11 4 items=["Grayscale (U8)", "Grayscale (I16)", "Grayscale (SGL)", "Complex (CSG)", "RGB (U32)", "HSL (U32)", "RGB (U64)"] ("Image Type")
        # "no wide angle camera found"
        n36 = call "IMAQ Create"("Image Name"=w66, "Image Type"=w59) -> ("New Image"=w62:T3)  [unwired: 3 in, 1 out]
        n37 = call "IMAQ SetImageSize"("Y Resolution"=120, "X Resolution"=320, "Image"=w62) -> ("Image Out"=w64:T3)  [unwired: 2 in, 1 out]
        n38 = call "IMAQ ImageToImage 2"("Image Src (Small)"=w63, "Image Src (Large)"=w64) -> ("Image Dst Out"=w65:T3)  [unwired: 8 in, 1 out]
      }
    }
    "Combined Camera Feed" <- w29
  }
  n39 = while {
    tunnel: w2 -> [_]
    stop <- FALSE stop-if-true
    # "Maintain LimeLight connection"
    n40 = local read "Enable_Streaming_GUI"() -> (w71:bool)
    n41 = Wait (ms)(milliseconds to wait=u32 1000) -> ()  [unwired: 1 out]
    n42 = case shown="True" w71 {
      frame False {
      }
      frame True {
        w89 = "320x240 MJPEG 22 fps" ("String")
        w88 = "/CameraPublisher/limelight/"
        # "manually configure the NT for a single LimeLight\ncamera in order to bypass WPILib's camera\nauto-detection which fails when the NTs are refreshed\nafter the code restarts on the roboRIO"
        n43 = case shown="False" "Camera Switch\nCamera Switch" {
          tunnel: ["11" "12"] -> w74
          frame False {
          }
          frame True {
          }
        }
        n44 = Concatenate Strings("10.42.65.", w74, ":5800") -> (w78:string)
        n45 = Concatenate Strings("mjpg:http://", w78) -> (w79:string)
        n46 = Concatenate Strings("ip:http://", w78) -> (w91:string)
        n47 = Build Array(w79, w79) -> (w93:string[])
        n48 = Concatenate Strings(w88, "source") -> (w90:string)
        n49 = Concatenate Strings(w88, "description") -> (w94:string)
        n50 = Concatenate Strings(w88, "mode") -> (w95:string)
        n51 = Build Array(w89) -> (w97:string[])
        n52 = Concatenate Strings(w88, "streams") -> (w92:string)
        n53 = Concatenate Strings(w88, "modes") -> (w96:string)
        n54 = call-poly <vilib>:"NT Write Value.vi"("value"=w91, "name"=w90) -> ()  [unwired: 9 in, 1 out]
        n55 = call-poly <vilib>:"NT Write Value.vi"("value"="limelight" ("String"), "name"=w94) -> ()  [unwired: 9 in, 1 out]
        n56 = call-poly <vilib>:"NT Write Value.vi"("value"=w89, "name"=w95) -> ()  [unwired: 9 in, 1 out]
        n57 = call-poly <vilib>:"NT Write Value.vi"("value"=w93, "name"=w92) -> ()  [unwired: 9 in, 1 out]
        n58 = call-poly <vilib>:"NT Write Value.vi"("value"=w97, "name"=w96) -> ()  [unwired: 9 in, 1 out]
      }
    }
  }
  n59 = while {
    tunnel: w4 -> [w102]
    stop <- FALSE stop-if-true
    # "Primary Indicators and Controls"
    n60 = Wait (ms)(milliseconds to wait=u32 50) -> ()  [unwired: 1 out]
    n61 = call <vilib>:"WPI_DashboardRetrieveStatusInfo.vi"("Window Mode Notifier"=w102, "TCP Cnx"="TCP") -> ("Power and Errors"=w105:T18, "Robot Metrics"=w107:T19, "Status Info"=w108:T20, "Control Info"=w106:T21, "Robot Mode"=w104:T7)  [unwired: 4 in, 1 out]
    "Mode" <- w104
    n62 = case shown="True" TRUE {
      tunnel: w108 -> [_ w112]
      tunnel: w107 -> [_ w111]
      tunnel: w106 -> [_ w113]
      tunnel: w105 -> [_ w110]
      tunnel: w104 -> [_ _]
      frame False {
      }
      frame True {
        n63 = stacked-sequence {
          tunnel: w113 -> [_ _ _ _ _ _ _ _ _ _ _ _]
          tunnel: w112 -> [w128 _ _ _ _ _ _ _ _ _ _ _]
          tunnel: w111 -> [_ _ _ _ _ _ _ _ _ _ _ _]
          tunnel: w110 -> [_ _ _ _ _ _ _ _ _ _ _ _]
          frame #0 {
            w118 = u32 1000  # (ms)
            # "general reporting"
            # "resource utilization"
            # "autonomous reporting"
            # "report robot status and resource utilization"
            n64 = Unbundle By Name(w128) -> ("Battery V"=→"Battery_Voltage_GUI":dbl)
            n65 = call-poly <vilib>:"NT Read Value.vi"("name"="Swerve_Output_Loop_Time" ("Name")) -> ("value"=w116:dbl)  [unwired: 8 in, 2 out]
            n66 = call-poly <vilib>:"NT Read Value.vi"("default value"=FALSE, "name"="Code_is_Running" ("Name")) -> ("value"=w121:bool)  [unwired: 7 in, 2 out]
            n67 = call-poly <vilib>:"NT Read Value.vi"("name"="Battery_Critical" ("Name")) -> ("value"=→"Battery_Critical_GUI":bool)  [unwired: 8 in, 2 out]
            n68 = call-poly <vilib>:"NT Read Value.vi"("name"="Diverting_Power" ("Name")) -> ("value"=→"Diverting_Power_GUI":bool)  [unwired: 8 in, 2 out]
            n69 = call-poly <vilib>:"NT Read Value.vi"("name"="Electrical_Fault" ("Name")) -> ("value"=→"Electrical_Fault_GUI":bool)  [unwired: 8 in, 2 out]
            n70 = call-poly <vilib>:"NT Read Value.vi"("name"="CAN_Bus_Fault" ("Name")) -> ("value"=→"CAN_Bus_Fault_GUI":bool)  [unwired: 8 in, 2 out]
            n71 = call-poly <vilib>:"NT Read Value.vi"("name"="Control_Latency_Alarm" ("Name")) -> ("value"=w157:bool)  [unwired: 8 in, 2 out]
            "Slow_Loop" <- w157
            n72 = call-poly <vilib>:"NT Read Value.vi"("name"="Control_Loop_Time" ("Name")) -> ("value"=w148:dbl)  [unwired: 8 in, 2 out]
            n73 = call-poly <vilib>:"NT Read Value.vi"("name"="Pose_Loop_Time" ("Name")) -> ("value"=w158:dbl)  [unwired: 8 in, 2 out]
            n74 = call-poly <vilib>:"NT Read Value.vi"("name"="Compressor_On" ("Name")) -> ("value"=→"Compressor_On_GUI":bool)  [unwired: 8 in, 2 out]
            n75 = call-poly <vilib>:"NT Read Value.vi"("name"="Pressure_Vent" ("Name")) -> ("value"=→"Pressure_Vent_GUI":bool)  [unwired: 8 in, 2 out]
            n76 = call-poly <vilib>:"NT Read Value.vi"("name"="Pressure_Transducer" ("Name")) -> ("value"=→"Pressure_Transducer_GUI":dbl)  [unwired: 8 in, 2 out]
            n77 = call-poly <vilib>:"NT Read Value.vi"("name"="Pressure_Leak" ("Name")) -> ("value"=→"Pressure_Leak_GUI":bool)  [unwired: 8 in, 2 out]
            n78 = To Unsigned Long Integer(number=w116) -> (unsigned 32bit integer=→"Swerve_Output_Loop_Time_GU":u32)
            n79 = To Unsigned Long Integer(number=w158) -> (unsigned 32bit integer=→"Pose_Loop_Time_GUI":u32)
            n80 = Not(x=w121) -> (.not. x?=w120:bool)
            n81 = To Unsigned Long Integer(number=w148) -> (unsigned 32bit integer=→"Control_Loop_Time_GUI":u32)
            n82 = call "Timer.vi"("Reset Timer"=w120) -> ("Time (ms)"=w119:u32)
            n83 = Greater?(x=w119, y=w118) -> (0:w117:bool)
            n84 = Select(t=u32 16711680 ("Numeric Text.Text Colors:Text Color"), s=w157, f=u32 4934475 ("Numeric Text.Text Colors:Text Color")) -> (s? t:f=w152:u32)
            n85 = global write "GlobalDashboard.vi" "Code_is_Running"(w117) -> ()
            n86 = property on="Control_Loop_Time_GUI" class="DigNum (strict)"("NumText.BG Color"=w152) -> ()  [unwired: 2 in, 2 out]
            n87 = call-poly <vilib>:"NT Read Value.vi"("name"="Auto_Error" ("Name")) -> ("value"=→"Auto_Error_GUI":bool)  [unwired: 8 in, 2 out]
            n88 = call-poly <vilib>:"NT Read Value.vi"("name"="Robot_is_Autonomous" ("Name")) -> ("value"=→"Robot_is_Autonomous_GUI_0" →"Robot_is_Autonomous_GUI_1" →"Robot_is_Autonomous_GUI_2":bool)  [unwired: 8 in, 2 out]
            n89 = local read "Dashboard Tab"() -> (w124:T1)
            n90 = local read "Dashboard Tab"() -> (w125:T1)
            n91 = case shown="\"Setup/Auto\"" w124 {
              frame "Checklist", Default {
              }
              frame "Setup/Auto" {
                n92 = call-poly <vilib>:"NT Read Value.vi"("default value"="No robot code versioning information..." ("Default Value"), "name"="Robot_Code_Version" ("Name")) -> ("value"=→"Robot_Code_Version_GUI":string)  [unwired: 7 in, 2 out]
              }
            }
            n93 = To Double Precision Float(number=w125) -> (double precision float=w126:dbl)
            n94 = call "ReducedBWSendToNT.vim"("Value In"=w126, "NT Name"="Dashboard_Tab" ("Name")) -> ()  [unwired: 1 out]
          }
          frame #1 {
            w166 = dbl[] [] ("default value")
            # "targeting data"
            # "report robot pose and targeting data"
            n95 = call-poly <vilib>:"NT Read Value.vi"("default value"=0.0, "name"="Alliance_Color" ("Name")) -> ("value"=w186:dbl)  [unwired: 7 in, 2 out]
            n96 = To Unsigned Word Integer(number=w186) -> (unsigned 16bit integer=w184:u16)
            n97 = call-poly <vilib>:"NT Read Value.vi"("name"="Alliance_Color" ("Name")) -> ("value"=w204:dbl)  [unwired: 8 in, 2 out]
            n98 = To Unsigned Word Integer(number=w204) -> (unsigned 16bit integer=w212:u16)
            n99 = Equal?(x=w184, y=WPI_DriverStationAllianceInfo."Red" ("x")) -> (x = y?=w177:bool)
            n100 = feedback #1(w212) -> (w208:u16)
            n101 = feedback-in #1(w212) -> ()
            n102 = Not Equal?(x=w212, y=w208) -> (x != y?=w210:bool)
            n103 = feedback #2("Field Map") -> (w213:u16)
            n104 = feedback-in #2("Field Map") -> ()
            n105 = Not Equal?(x="Field Map", y=w213) -> (x != y?=w215:bool)
            n106 = call-poly <vilib>:"NT Read Value.vi"("default value"=300.0 ("Default Value"), "name"="Field_Width" ("Name")) -> ("value"=w178:dbl)  [unwired: 7 in, 2 out]
            n107 = call-poly <vilib>:"NT Read Value.vi"("default value"=600.0 ("Default Value"), "name"="Field_Length" ("Name")) -> ("value"=w179:dbl)  [unwired: 7 in, 2 out]
            n108 = Select(t=u32 16711680 ("Color"), s=w177, f=u32 255 ("Color")) -> (s? t:f=w180:u32)
            n109 = First Call?() -> (First Call?: T/F=w209:bool)
            n110 = call "EdgeTrigger.vi"("Input Signal"="Export_Robot_Pose") -> ("Rising Edge Trigger"=w216:bool)  [unwired: 2 out]
            n111 = stacked-sequence {
              tunnel: w180 -> [w228 w230 w233]
              frame #0 {
                w229 = u32 0 ("Active Plot")
                n112 = property on="Robot Pose 2" class="XYGraph (strict)"("Active Plot"=w229, "Plot.Plot Color"=w228) -> ()  [unwired: 2 in, 2 out]
                n113 = property on="Robot Pose 1" class="XYGraph (strict)"("Active Plot"=w229, "Plot.Plot Color"=w228) -> ()  [unwired: 2 in, 2 out]
              }
              frame #1 {
                w231 = u32 1 ("Active Plot")
                n114 = property on="Robot Pose 2" class="XYGraph (strict)"("Active Plot"=w231, "Plot.Plot Color"=w230) -> ()  [unwired: 2 in, 2 out]
                n115 = property on="Robot Pose 1" class="XYGraph (strict)"("Active Plot"=w231, "Plot.Plot Color"=w230) -> ()  [unwired: 2 in, 2 out]
              }
              frame #2 {
                w232 = u32 5 ("Active Plot")
                n116 = property on="Robot Pose 2" class="XYGraph (strict)"("Active Plot"=w232, "Plot.Fill/Pt. Color"=w233) -> ()  [unwired: 2 in, 2 out]
                n117 = property on="Robot Pose 1" class="XYGraph (strict)"("Active Plot"=w232, "Plot.Fill/Pt. Color"=w233) -> ()  [unwired: 2 in, 2 out]
              }
            }
            n118 = Compound Arithmetic op=OR(w210, w209, w215) -> (w211:bool)
            n119 = case shown="True" w211 {
              tunnel: w212 -> [_ w240]
              tunnel: "Field Map" -> [_ w238]
              frame False {
              }
              frame True {
                # "load and display a field map"
                n120 = To Long Integer(number=w238) -> (32bit integer=w236:i32)
                n121 = Current VI's Path() -> (path=w243:path)
                n122 = Strip Path(path=w243) -> (stripped path=w242:path)  [unwired: 1 out]
                n123 = Strip Path(path=w242) -> (stripped path=w239:path)  [unwired: 1 out]
                n124 = List Folder(path=w239, pattern="*map*.png") -> (filenames=w237:string[])  [unwired: 2 in, 3 out]
                n125 = Index Array(array=w237, index=w236) -> (element=w235:string)
                n126 = property on="Field Map" class="Ring (strict)"("Strings []"=w237) -> ()  [unwired: 2 in, 2 out]
                n127 = Build Path(base path=w239, name or relative path=w235) -> (appended path=w241:path)
                n128 = call <vilib>:"Read PNG File.vi"("path to PNG file"=w241) -> ("error out"=w245:errorcluster, "image data"=w244:T22)  [unwired: 8 in, 1 out]
                n129 = case shown="No Error" w245 {
                  tunnel: w244 -> [w248 _]
                  tunnel: w240 -> [w263 _]
                  frame No Error {
                    w258 = T11 4 items=["Grayscale (U8)", "Grayscale (I16)", "Grayscale (SGL)", "Complex (CSG)", "RGB (U32)", "HSL (U32)", "RGB (U64)", "Grayscale (U16)"] ("Image Type")
                    w278 = T11 4 items=["Grayscale (U8)", "Grayscale (I16)", "Grayscale (SGL)", "Complex (CSG)", "RGB (U32)", "HSL (U32)", "RGB (U64)", "Grayscale (U16)"] ("Image Type")
                    n130 = call <vilib>:"Unflatten Pixmap.vi"("image data"=w248) -> ("24-bit pixmap"=w277:u32[][])  [unwired: 4 in, 6 out]
                    n131 = call <vilib>:"Unflatten Pixmap.vi"("image data"=w248) -> ("24-bit pixmap"=w257:u32[][])  [unwired: 4 in, 6 out]
                    n132 = property on="Robot Pose 1" class="XYGraph (strict)"() -> ("Width"=w281:u32, "Height"=w280:u32)  [unwired: 2 in, 2 out]
                    n133 = property on="Robot Pose 2" class="XYGraph (strict)"() -> ("Width"=w261:u32, "Height"=w260:u32)  [unwired: 2 in, 2 out]
                    n134 = call "IMAQ Create"("Image Name"="field1", "Image Type"=w278) -> ("New Image"=w276:T3)  [unwired: 3 in, 1 out]
                    n135 = call "IMAQ Create"("Image Name"="field2", "Image Type"=w258) -> ("New Image"=w256:T3)  [unwired: 3 in, 1 out]
                    n136 = Equal?(x=w263, y=WPI_DriverStationAllianceInfo."Red" ("x")) -> (x = y?=w265:bool)
                    n137 = call "IMAQ ArrayToColorImage"("Image Pixels (U32)"=w277, "Image"=w276) -> ("Image Out"=w275:T3)  [unwired: 3 in, 1 out]
                    n138 = call "IMAQ ArrayToColorImage"("Image Pixels (U32)"=w257, "Image"=w256) -> ("Image Out"=w255:T3)  [unwired: 3 in, 1 out]
                    n139 = To Long Integer(number=w281) -> (32bit integer=w271:i32)
                    n140 = To Long Integer(number=w280) -> (32bit integer=w272:i32)
                    n141 = To Long Integer(number=w261) -> (32bit integer=w251:i32)
                    n142 = To Long Integer(number=w260) -> (32bit integer=w252:i32)
                    n143 = call "IMAQ Resample"("X Resolution"=w271, "Y Resolution"=w272, "Image Src"=w275) -> ("Image Dst Out"=w270:T3)  [unwired: 7 in, 1 out]
                    n144 = call "IMAQ Resample"("X Resolution"=w251, "Y Resolution"=w252, "Image Src"=w255) -> ("Image Dst Out"=w250:T3)  [unwired: 7 in, 1 out]
                    n145 = Select(t=180.0, s=w265, f=0.0) -> (s? t:f=w268:dbl)
                    n146 = To Single Precision Float(number=w268) -> (single precision float=w246:sgl)
                    n147 = call "IMAQ Rotate"("Angle (degrees)"=w246, "Image Src"=w270) -> ("Image Dst Out"=w269:T3)  [unwired: 8 in, 1 out]
                    n148 = call "IMAQ Rotate"("Angle (degrees)"=w246, "Image Src"=w250) -> ("Image Dst Out"=w249:T3)  [unwired: 8 in, 1 out]
                    n149 = call "IMAQ ColorImageToArray"("Image"=w269) -> ("Image Pixels (U32)"=w274:u32[][])  [unwired: 3 in, 2 out]
                    n150 = call "IMAQ ColorImageToArray"("Image"=w249) -> ("Image Pixels (U32)"=w254:u32[][])  [unwired: 3 in, 2 out]
                    n151 = call <vilib>:"Flatten Pixmap.vi"("24-bit pixmap"=w274) -> ("image data"=w273:T22)  [unwired: 10 in]
                    n152 = call <vilib>:"Flatten Pixmap.vi"("24-bit pixmap"=w254) -> ("image data"=w253:T22)  [unwired: 10 in]
                    n153 = call <vilib>:"Draw Flattened Pixmap.vi"("image data"=w273) -> ("new picture"=w262:picture)  [unwired: 8 in]
                    n154 = call <vilib>:"Draw Flattened Pixmap.vi"("image data"=w253) -> ("new picture"=w247:picture)  [unwired: 8 in]
                    n155 = property on="Robot Pose 1" class="XYGraph (strict)"("PlotImages.Back"=w262) -> ()  [unwired: 2 in, 2 out]
                    n156 = property on="Robot Pose 2" class="XYGraph (strict)"("PlotImages.Back"=w247) -> ()  [unwired: 2 in, 2 out]
                  }
                  frame Error {
                  }
                }
              }
            }
            n157 = case shown="True" w216 {
              frame False {
              }
              frame True {
                # "export the current robot pose data"
                n158 = Get Date/Time In Seconds() -> (seconds since 1Jan1904=w295:timestamp)
                n159 = Format Date/Time String(time format string (%c)="%Y-%m-%d_%H-%M", seconds (now)=w295) -> (date/time string=w293:string)  [unwired: 1 in]
                n160 = Concatenate Strings("robot pose data " ("string"), w293) -> (w291:string)
                n161 = Current VI's Path() -> (path=w290:path)
                n162 = String To Path(string=w291) -> (path=w287:path)
                n163 = Strip Path(path=w290) -> (stripped path=w289:path)  [unwired: 1 out]
                n164 = Strip Path(path=w289) -> (stripped path=w288:path)  [unwired: 1 out]
                n165 = Build Path(base path=w288, name or relative path=w287) -> (appended path=w286:path)
                n166 = invoke on="Robot Pose 1" class="XYGraph (strict)" method="Export Image"("FileType"=enum32{"BMP", "EPS", "EMF", "PICT"}."BMP" ("File Type"), "Target"=enum32{"File", "Clipboard"}."File", "Path"=w286, "HideGrid"=TRUE ("Hide Grid"), "Overwrite"=TRUE ("Always Overwrite")) -> ()  [unwired: 3 in, 8 out]
              }
            }
            n167 = property on="Robot Pose 1" class="XYGraph (strict)"("XScale.Maximum"=w178, "YScale.Maximum"=w179) -> ()  [unwired: 2 in, 2 out]
            n168 = property on="Robot Pose 2" class="XYGraph (strict)"("XScale.Maximum"=w178, "YScale.Maximum"=w179) -> ()  [unwired: 2 in, 2 out]
            n169 = call-poly <vilib>:"NT Read Value.vi"("default value"=0.0 ("Default Value"), "name"="Robot_H" ("Name")) -> ("value"=w227:dbl)  [unwired: 7 in, 2 out]
            n170 = call-poly <vilib>:"NT Read Value.vi"("default value"=-1.0 ("Default Value"), "name"="Robot_Y" ("Name")) -> ("value"=w176:dbl)  [unwired: 7 in, 2 out]
            "Robot_Y" <- w176
            n171 = call-poly <vilib>:"NT Read Value.vi"("default value"=-1.0 ("Default Value"), "name"="Robot_X" ("Name")) -> ("value"=w175:dbl)  [unwired: 7 in, 2 out]
            "Robot_X" <- w175
            n172 = call-poly <vilib>:"NT Read Value.vi"("default value"=30.0 ("Default Value"), "name"="Robot_Width_Bumpers" ("Name")) -> ("value"=w198:dbl)  [unwired: 7 in, 2 out]
            n173 = call-poly <vilib>:"NT Read Value.vi"("default value"=30.0 ("Default Value"), "name"="Robot_Length_Bumpers" ("Name")) -> ("value"=w199:dbl)  [unwired: 7 in, 2 out]
            n174 = Quotient & Remainder(x=w227, y=360.0) -> (x-y*floor(x/y)=→"Robot_H_GUI":dbl)  [unwired: 1 out]
            n175 = call-poly <vilib>:"NT Read Value.vi"("default value"=w166, "name"="Auto_Path_Xs" ("Name")) -> ("value"=w167:dbl[])  [unwired: 7 in, 2 out]
            n176 = call-poly <vilib>:"NT Read Value.vi"("default value"=w166, "name"="Auto_Path_Ys" ("Name")) -> ("value"=w169:dbl[])  [unwired: 7 in, 2 out]
            n177 = Bundle("value"=w169, "value"=w167) -> (w171:cluster{"value":dbl[], "value":dbl[]})  [unwired: 1 in]
            n178 = call "RenderRobotPose.vi"("Robot X (in)"=w175, "Robot Width (in)"=w198, "Robot Length (in)"=w199, "Buffer Time (min)"=0.5, "Robot Y (in)"=w176, "Robot Heading (deg)"=w227, "Planned Path"=w171, "Robot Enabled"=TRUE, "Reset"="Clear_Robot_Pose_Display") -> ("Robot Pose"=→"Robot Pose 2" →"Robot Pose 1":cluster{dbl[], dbl[]}[])  [unwired: 6 in]
            n179 = local read "No_Secondary_Camera"() -> (w192:bool)
            n180 = property on="Robot Pose 2" class="XYGraph (strict)"("Visible"=w192) -> ()  [unwired: 2 in, 2 out]
            n181 = call-poly <vilib>:"NT Read Value.vi"("name"="Lemon_Vision_Fault" ("Name")) -> ("value"=→"(Front) Lemon_Vision_Fault_GUI":bool)  [unwired: 8 in, 2 out]
            n182 = call-poly <vilib>:"NT Read Value.vi"("name"="LL_Valid" ("Name")) -> ("value"=→"LL_Valid":bool)  [unwired: 8 in, 2 out]
            n183 = call-poly <vilib>:"NT Read Value.vi"("name"="Lime_Vision_Fault" ("Name")) -> ("value"=→"(Back) Lime_Vision_Fault_GUI":bool)  [unwired: 8 in, 2 out]
            n184 = call-poly <vilib>:"NT Read Value.vi"("default value"=0.0, "name"="Distance_to_Target" ("Name")) -> ("value"=→"Distance_to_Target":dbl)  [unwired: 7 in, 2 out]
          }
          frame #2 {
            # "driver control configuration"
            # "robot configuration"
            # "robot and driver control configuration"
            n185 = local read "Dashboard Tab"() -> (w297:T1)
            n186 = case shown="\"Setup/Auto\"" w297 {
              frame "Checklist", Default {
              }
              frame "Setup/Auto" {
                n187 = call-poly <vilib>:"NT Read Value.vi"("default value"="No robot profile..." ("Default Value"), "name"="Robot_Profile" ("Name")) -> ("value"=→"Robot_Profile_GUI":string)  [unwired: 7 in, 2 out]
              }
            }
            n188 = Build Array("N/A") -> (w308:string[])
            n189 = And(x="Calibrate_Joysticks_GUI", y="Arm_Calibrate_Joysticks") -> (x .and. y?=w298:bool)
            n190 = To Double Precision Float(number="Select Driver Profile") -> (double precision float=w301:dbl)
            n191 = call-poly <vilib>:"NT Read Value.vi"("default value"=w308, "name"="Legal_Drivers" ("Name")) -> ("value"=w307:string[])  [unwired: 7 in, 2 out]
            "Legal_Drivers_GUI" <- w307
            n192 = Not(x="Arm_Calibrate_Joysticks") -> (.not. x?=w310:bool)
            n193 = call "ReducedBWSendToNT.vim"("Value In"=w301, "NT Name"="Selected_Driver" ("Name")) -> ()  [unwired: 1 out]
            n194 = property on="Select Driver Profile" class="Ring (strict)"("Strings []"=w307) -> ()  [unwired: 2 in, 2 out]
            n195 = call "ReducedBWSendToNT.vim"("Value In"=w298, "NT Name"="Calibrate_Joysticks" ("Name")) -> ()  [unwired: 1 out]
            n196 = Select(t=cluster{u32, u32}[] [{11776947, 16448250}, {16448250, 16448250}] ("Colors [4]"), s=w310, f=cluster{u32, u32}[] [{6618880, 16448250}, {16448250, 16448250}] ("Colors [4]")) -> (s? t:f=w311:cluster{u32, u32}[])
            n197 = property on="Calibrate_Joysticks_GUI" class="Bool"("Colors [4]"=w311) -> ()  [unwired: 2 in, 2 out]
            n198 = case shown="True" "Launch_Camera" {
              frame False {
              }
              frame True {
                n199 = call <vilib>:"System Exec.vi"("command line"="\"C:\\Program Files\\Google\\Chrome\\Application\\chrome.exe\" --load-extension=\"C:\\cameraExtension\" --new-window \"http://roborio-4265-frc.local:1181/\" --user-data-dir=\"C:\\cameraExtension\\UserData\"") -> ()  [unwired: 7 in, 4 out]
              }
            }
          }
          frame #3 {
            # "configure auto play"
            # "set robot pose"
            # "autonomous configuration"
            n200 = call "ReducedBWSendToNT.vim"("Value In"="Manual_Start_X", "NT Name"="Manual_Start_X" ("Name")) -> ()  [unwired: 1 out]
            n201 = call "ReducedBWSendToNT.vim"("Value In"="Manual_Start_Y", "NT Name"="Manual_Start_Y" ("Name")) -> ()  [unwired: 1 out]
            n202 = call "ReducedBWSendToNT.vim"("Value In"="Manual_Start_H", "NT Name"="Manual_Start_H" ("Name")) -> ()  [unwired: 1 out]
            n203 = call "ReducedBWSendToNT.vim"("Value In"="Disable_Fusion_While_Autonomous", "NT Name"="Disable_Fusion_While_Autonomous" ("Name")) -> ()  [unwired: 1 out]
            n204 = call "ReducedBWSendToNT.vim"("Value In"="Disable_Fusion_While_Disabled", "NT Name"="Disable_Fusion_While_Disabled" ("Name")) -> ()  [unwired: 1 out]
            n205 = call "ReducedBWSendToNT.vim"("Value In"="Push_Robot_Start_GUI", "NT Name"="Push_Robot_Start" ("Name")) -> ()  [unwired: 1 out]
            n206 = local read "Dashboard Tab"() -> (w319:T1)
            n207 = To Double Precision Float(number="Select Autonomous Play") -> (double precision float=w322:dbl)
            n208 = call "ReducedBWSendToNT.vim"("Value In"="Auto_Test_Mode_GUI", "NT Name"="Auto_Test_Mode" ("Name")) -> ()  [unwired: 1 out]
            n209 = call "ReducedBWSendToNT.vim"("Value In"="Auto_Delay_GUI", "NT Name"="Auto_Delay" ("Name")) -> ()  [unwired: 1 out]
            n210 = call "ReducedBWSendToNT.vim"("Value In"="Force_Human_Control_GUI", "NT Name"="Force_Human_Control" ("Name")) -> ()  [unwired: 1 out]
            n211 = call "ReducedBWSendToNT.vim"("Value In"=w322, "NT Name"="Selected_Auto_Play" ("Name")) -> ()  [unwired: 1 out]
            n212 = call "ReducedBWSendToNT.vim"("Value In"="Refresh_Auto_Play_List_GUI", "NT Name"="Refresh_Auto_Play_List" ("Name")) -> ()  [unwired: 1 out]
            n213 = case shown="\"Setup/Auto\"" w319 {
              tunnel: "Select Autonomous Play" -> [_ w342]
              tunnel: "Refresh_Auto_Play_List_GUI" -> [_ w341]
              frame "Checklist", Default {
              }
              frame "Setup/Auto" {
                w359 = "N/A" ("Default Value")
                n214 = call-poly <vilib>:"NT Read Value.vi"("default value"=0.0, "name"="Suggested_Start_H" ("Name")) -> ("value"=w358:dbl)  [unwired: 7 in, 2 out]
                n215 = call-poly <vilib>:"NT Read Value.vi"("default value"=0.0, "name"="Suggested_Start_X" ("Name")) -> ("value"=w356:dbl)  [unwired: 7 in, 2 out]
                n216 = call-poly <vilib>:"NT Read Value.vi"("default value"=0.0, "name"="Suggested_Start_Y" ("Name")) -> ("value"=w357:dbl)  [unwired: 7 in, 2 out]
                n217 = Build Array("N/A") -> (w362:string[])
                n218 = call "Is Value Changed.vim"("value"=w342) -> ("changed or first call?"=w343:bool)
                n219 = call "Is Value Changed.vim"("value"=w358) -> ("changed or first call?"=w349:bool)
                n220 = call "Is Value Changed.vim"("value"=w356) -> ("changed or first call?"=w345:bool)
                n221 = call "Is Value Changed.vim"("value"=w357) -> ("changed or first call?"=w347:bool)
                n222 = call-poly <vilib>:"NT Read Value.vi"("default value"=w359, "name"="Auto_Playbook" ("Name")) -> ("value"=→"Auto_Playbook_GUI":string)  [unwired: 7 in, 2 out]
                n223 = call-poly <vilib>:"NT Read Value.vi"("default value"=w359, "name"="Auto_Path_Suffix" ("Name")) -> ("value"=→"Auto_Suffix_GUI":string)  [unwired: 7 in, 2 out]
                n224 = call-poly <vilib>:"NT Read Value.vi"("default value"=w362, "name"="Legal_Auto_Plays" ("Name")) -> ("value"=w363:string[])  [unwired: 7 in, 2 out]
                n225 = Compound Arithmetic op=OR(w343, w341, w345) -> (w344:bool)
                n226 = Compound Arithmetic op=OR(w343, w341, w347) -> (w346:bool)
                n227 = Compound Arithmetic op=OR(w343, w341, w349) -> (w348:bool)
                n228 = property on="Select Autonomous Play" class="Ring (strict)"("Strings []"=w363) -> ()  [unwired: 2 in, 2 out]
                n229 = case shown="True" w348 {
                  tunnel: w358 -> [_ w368]
                  frame False {
                  }
                  frame True {
                    n230 = property on="Manual_Start_H" class="DigNum (strict)"("Value"=w368) -> ()  [unwired: 2 in, 2 out]
                  }
                }
                n231 = case shown="True" w346 {
                  tunnel: w357 -> [_ w369]
                  frame False {
                  }
                  frame True {
                    n232 = property on="Manual_Start_Y" class="DigNum (strict)"("Value"=w369) -> ()  [unwired: 2 in, 2 out]
                  }
                }
                n233 = case shown="True" w344 {
                  tunnel: w356 -> [_ w370]
                  frame False {
                  }
                  frame True {
                    n234 = property on="Manual_Start_X" class="DigNum (strict)"("Value"=w370) -> ()  [unwired: 2 in, 2 out]
                  }
                }
              }
            }
          }
          frame #4 {
            w396 = bool[] [FALSE, FALSE, FALSE, FALSE, FALSE, FALSE] ("default value")
            w395 = bool[] [FALSE, FALSE, FALSE, FALSE, FALSE, FALSE] ("Default Value")
            w382 = cluster{u32, u32}[] [{9567230, 16448250}, {16448250, 16448250}] ("Un-selected Color")
            # "master state controller"
            # "state indicators"
            n235 = global read "GlobalDashboard.vi" "Code_is_Running"() -> (w394:bool)
            n236 = call-poly <vilib>:"NT Read Value.vi"("default value"=w396, "name"="Confirmed_States" ("Name")) -> ("value"=w391:bool[])  [unwired: 7 in, 2 out]
            n237 = call-poly <vilib>:"NT Read Value.vi"("default value"=w395, "name"="Disallowed_States" ("Name")) -> ("value"=w393:bool[])  [unwired: 7 in, 2 out]
            n238 = Select(t=w393, s=w394, f=w395) -> (s? t:f=w392:bool[])
            n239 = Select(t=w391, s=w394, f=w396) -> (s? t:f=w390:bool[])
            n240 = Index Array(array=w392) -> (element #1=w375:bool, element #2=w374:bool, element #3=w373:bool, element #4=w372:bool, element #5=w371:bool)  [unwired: 5 in]
            n241 = Index Array(array=w390) -> (element #1=w380:bool, element #2=w379:bool, element #3=w378:bool, element #4=w377:bool, element #5=w376:bool)  [unwired: 5 in]
            "State_AMP" <- w378
            "State_Climbing" <- w377
            n242 = call "ButtonColorChooser.vi"("Un-selected Color"=w382, "Disallowed"=w375, "Confirmed"=w380) -> ("Final Color"=w383:cluster{u32, u32}[])  [unwired: 8 in]
            n243 = call "ButtonColorChooser.vi"("Un-selected Color"=w382, "Disallowed"=w374, "Confirmed"=w379) -> ("Final Color"=w400:cluster{u32, u32}[])  [unwired: 8 in]
            n244 = call "ButtonColorChooser.vi"("Un-selected Color"=w382, "Disallowed"=w373, "Confirmed"=w378) -> ("Final Color"=w386:cluster{u32, u32}[])  [unwired: 8 in]
            n245 = call "ButtonColorChooser.vi"("Un-selected Color"=w382, "Disallowed"=w372, "Confirmed"=w377) -> ("Final Color"=w385:cluster{u32, u32}[])  [unwired: 8 in]
            n246 = call "ButtonColorChooser.vi"("Un-selected Color"=w382, "Disallowed"=w371, "Confirmed"=w376) -> ("Final Color"=w384:cluster{u32, u32}[])  [unwired: 8 in]
            n247 = property on="Master_State_STOW_Indicator" class="Bool (strict)"("Colors [4]"=w383) -> ()  [unwired: 2 in, 2 out]
            n248 = property on="Master_State_SPEAKER_Indicator" class="Bool (strict)"("Colors [4]"=w400) -> ()  [unwired: 2 in, 2 out]
            n249 = property on="Master_State_AMP_Indicator" class="Bool (strict)"("Colors [4]"=w386) -> ()  [unwired: 2 in, 2 out]
            n250 = property on="Master_State_CLIMB_Indicator" class="Bool (strict)"("Colors [4]"=w385) -> ()  [unwired: 2 in, 2 out]
            n251 = property on="Master_State_TRAP_Indicator" class="Bool (strict)"("Colors [4]"=w384) -> ()  [unwired: 2 in, 2 out]
            "Master_State_SPEAKER_Indicator" <- FALSE ("Master_State_0_Indicator")
            "Master_State_AMP_Indicator" <- FALSE ("Master_State_0_Indicator")
            "Master_State_CLIMB_Indicator" <- FALSE ("Master_State_0_Indicator")
            "Master_State_TRAP_Indicator" <- FALSE ("Master_State_0_Indicator")
            "Master_State_STOW_Indicator" <- FALSE ("Master_State_STOW_Indicator")
          }
          frame #5 {
            # "actuator test interlocks"
            # "emergency overrides"
            # "emergency overrides and interlocks"
            n252 = global read "GlobalDashboard.vi" "Code_is_Running"() -> (w404:bool)
            n253 = call-poly <vilib>:"NT Read Value.vi"("default value"=FALSE, "name"="Robot_in_Safety_Override" ("Name")) -> ("value"=w406:bool)  [unwired: 7 in, 2 out]
            n254 = call "EdgeTrigger.vi"("Input Signal"=w406) -> ("All Edge Trigger"=w407:bool)  [unwired: 2 out]
            n255 = call "EdgeTrigger.vi"("Input Signal"=w404) -> ("Falling Edge Trigger"=w403:bool)  [unwired: 2 out]
            n256 = call "ReducedBWSendToNT.vim"("Value In"="Clear_Errors_GUI", "NT Name"="Clear_Errors" ("Name")) -> ()  [unwired: 1 out]
            n257 = call "ReducedBWSendToNT.vim"("Value In"="Super_Test_Mode_GUI", "NT Name"="Super_Test_Mode" ("Name")) -> ()  [unwired: 1 out]
            n258 = call "ReducedBWSendToNT.vim"("Value In"="Auto_Targeting_Override", "NT Name"="Auto_Targeting_Override" ("Name")) -> ()  [unwired: 1 out]
            n259 = call "ReducedBWSendToNT.vim"("Value In"="Field_Oriented_Override_GUI", "NT Name"="Field_Oriented_Override" ("Name")) -> ()  [unwired: 1 out]
            n260 = case shown="True" w407 {
              tunnel: w406 -> [_ w430]
              frame False {
              }
              frame True {
                n261 = property on="Master_Safety_Override_1" class="Bool (strict)"("Value"=w430) -> ()  [unwired: 2 in, 2 out]
              }
            }
            n262 = case shown="True" w403 {
              frame False {
              }
              frame True {
                n263 = property on="Master_Safety_Override_1" class="Bool (strict)"("Value"=FALSE ("Master_Safety_Override_1")) -> ()  [unwired: 2 in, 2 out]
              }
            }
            n264 = call "ReducedBWSendToNT.vim"("Value In"="Master_Safety_Override_1", "NT Name"="Master_Safety_Override" ("Name")) -> ()  [unwired: 1 out]
            n265 = property on="Actuator Testing" class="Ring (strict)"() -> ("RingText.Text"=w416:string)  [unwired: 2 in, 2 out]
            n266 = Build Array("No_Test") -> (w428:string[])
            n267 = call "ReducedBWSendToNT.vim"("Value In"="Free_Tuning_Variable_GUI", "NT Name"="Free_Tuning_Variable" ("Name")) -> ()  [unwired: 1 out]
            n268 = call-poly <vilib>:"NT Read Value.vi"("default value"=w428, "name"="Legal_Actuator_Names" ("Name")) -> ("value"=w427:string[])  [unwired: 7 in, 2 out]
            n269 = call "ReducedBWSendToNT.vim"("Value In"=w416, "NT Name"="Test_Actuator_Name" ("Name")) -> ()  [unwired: 1 out]
            n270 = call "ReducedBWSendToNT.vim"("Value In"="Test_Actuator_Value_GUI", "NT Name"="Test_Actuator_Value" ("Name")) -> ()  [unwired: 1 out]
            n271 = call "ReducedBWSendToNT.vim"("Value In"="Test_Actuator_Period_GUI", "NT Name"="Test_Actuator_Period" ("Name")) -> ()  [unwired: 1 out]
            n272 = property on="Actuator Testing" class="Ring (strict)"("Strings []"=w427) -> ()  [unwired: 2 in, 2 out]
          }
          frame #6 {
            # "drivebase subsytem"
            n273 = call "SwerveModuleReadData.vi"("NT Name (Errors)"="Swerve_1_Errors", "NT Name (Details)"="Swerve_1_Details" ("NT Name (Tune)")) -> ("Shifter State"=→"Swerve_1_Shifter_State":string, "Drive Velocity"=→"Swerve_1_Drive_Velocity":dbl, "Drive Temperature"=→"Swerve_1_Drive_Temperature":dbl, "Azimuth Position"=→"Swerve_1_Azimuth_Position":dbl, "Drive Overheating"=w490:T23, "Drive Fault"=w444:T23, "Azimuth Fault"=w489:T23)  [unwired: 3 in]
            n274 = call "SwerveModuleReadData.vi"("NT Name (Errors)"="Swerve_0_Errors", "NT Name (Details)"="Swerve_0_Details" ("NT Name (Tune)")) -> ("Shifter State"=→"Swerve_0_Shifter_State":string, "Drive Velocity"=→"Swerve_0_Drive_Velocity":dbl, "Drive Temperature"=→"Swerve_0_Drive_Temperature":dbl, "Azimuth Position"=→"Swerve_0_Azimuth_Position":dbl, "Drive Overheating"=w500:T23, "Drive Fault"=w446:T23, "Azimuth Fault"=w496:T23)  [unwired: 3 in]
            n275 = call-poly <vilib>:"NT Read Value.vi"("name"="IMU_Failure" ("Name")) -> ("value"=→"IMU_Failure_GUI":bool)  [unwired: 8 in, 2 out]
            n276 = call-poly <vilib>:"NT Read Value.vi"("name"="Field_Oriented" ("Name")) -> ("value"=→"Field_Oriented_GUI":bool)  [unwired: 8 in, 2 out]
            n277 = call "SwerveModuleReadData.vi"("NT Name (Errors)"="Swerve_2_Errors", "NT Name (Details)"="Swerve_2_Details" ("NT Name (Tune)")) -> ("Shifter State"=→"Swerve_2_Shifter_State":string, "Drive Velocity"=→"Swerve_2_Drive_Velocity":dbl, "Drive Temperature"=→"Swerve_2_Drive_Temperature":dbl, "Azimuth Position"=→"Swerve_2_Azimuth_Position":dbl, "Drive Overheating"=w486:T23, "Drive Fault"=w442:T23, "Azimuth Fault"=w485:T23)  [unwired: 3 in]
            n278 = call "SwerveModuleReadData.vi"("NT Name (Errors)"="Swerve_3_Errors", "NT Name (Details)"="Swerve_3_Details" ("NT Name (Tune)")) -> ("Shifter State"=→"Swerve_3_Shifter_State":string, "Drive Velocity"=→"Swerve_3_Drive_Velocity":dbl, "Drive Temperature"=→"Swerve_3_Drive_Temperature":dbl, "Azimuth Position"=→"Swerve_3_Azimuth_Position":dbl, "Drive Overheating"=w482:T23, "Drive Fault"=w440:T23, "Azimuth Fault"=w481:T23)  [unwired: 3 in]
            n279 = Unbundle(w490) -> ("Boolean"=w479:bool, "Numeric Text.Text Colors:Text Color"=w477:u32)
            n280 = Unbundle(w489) -> ("Boolean"=w480:bool, "Numeric Text.Text Colors:Text Color"=w478:u32)
            n281 = Unbundle(w500) -> ("Boolean"=w498:bool, "Numeric Text.Text Colors:Text Color"=w499:u32)
            n282 = Unbundle(w496) -> ("Boolean"=w495:bool, "Numeric Text.Text Colors:Text Color"=w493:u32)
            n283 = Unbundle(w486) -> ("Boolean"=w471:bool, "Numeric Text.Text Colors:Text Color"=w469:u32)
            n284 = Unbundle(w446) -> ("Boolean"=w438:bool, "Numeric Text.Text Colors:Text Color"=w447:u32)
            n285 = Unbundle(w485) -> ("Boolean"=w472:bool, "Numeric Text.Text Colors:Text Color"=w470:u32)
            n286 = Unbundle(w482) -> ("Boolean"=w462:bool, "Numeric Text.Text Colors:Text Color"=w461:u32)
            n287 = Unbundle(w481) -> ("Boolean"=w463:bool, "Numeric Text.Text Colors:Text Color"=w464:u32)
            n288 = Unbundle(w444) -> ("Boolean"=w437:bool, "Numeric Text.Text Colors:Text Color"=w445:u32)
            n289 = Unbundle(w442) -> ("Boolean"=w436:bool, "Numeric Text.Text Colors:Text Color"=w443:u32)
            n290 = Unbundle(w440) -> ("Boolean"=w435:bool, "Numeric Text.Text Colors:Text Color"=w441:u32)
            n291 = property on="Swerve_3_Drive_Velocity" class="DigNum (strict)"("NumText.BG Color"=w441) -> ()  [unwired: 2 in, 2 out]
            n292 = property on="Swerve_0_Azimuth_Position" class="DigNum (strict)"("NumText.BG Color"=w493) -> ()  [unwired: 2 in, 2 out]
            n293 = property on="Swerve_0_Drive_Temperature" class="DigNum (strict)"("NumText.BG Color"=w499) -> ()  [unwired: 2 in, 2 out]
            n294 = property on="Swerve_1_Azimuth_Position" class="DigNum (strict)"("NumText.BG Color"=w478) -> ()  [unwired: 2 in, 2 out]
            n295 = property on="Swerve_1_Drive_Temperature" class="DigNum (strict)"("NumText.BG Color"=w477) -> ()  [unwired: 2 in, 2 out]
            n296 = property on="Swerve_2_Azimuth_Position" class="DigNum (strict)"("NumText.BG Color"=w470) -> ()  [unwired: 2 in, 2 out]
            n297 = property on="Swerve_2_Drive_Temperature" class="DigNum (strict)"("NumText.BG Color"=w469) -> ()  [unwired: 2 in, 2 out]
            n298 = property on="Swerve_3_Azimuth_Position" class="DigNum (strict)"("NumText.BG Color"=w464) -> ()  [unwired: 2 in, 2 out]
            n299 = property on="Swerve_3_Drive_Temperature" class="DigNum (strict)"("NumText.BG Color"=w461) -> ()  [unwired: 2 in, 2 out]
            n300 = property on="Swerve_0_Drive_Velocity" class="DigNum (strict)"("NumText.BG Color"=w447) -> ()  [unwired: 2 in, 2 out]
            n301 = property on="Swerve_2_Drive_Velocity" class="DigNum (strict)"("NumText.BG Color"=w443) -> ()  [unwired: 2 in, 2 out]
            n302 = property on="Swerve_1_Drive_Velocity" class="DigNum (strict)"("NumText.BG Color"=w445) -> ()  [unwired: 2 in, 2 out]
            n303 = call-poly <vilib>:"NT Read Value.vi"("name"="Using_Auto_Targeting" ("Name")) -> ("value"=→"Using_Auto_Targeting":bool)  [unwired: 8 in, 2 out]
            n304 = Build Array(w495, w480, w472, w463) -> (→"Swerve_Azimuth_Fault_Array":bool[])
            n305 = Build Array(w498, w479, w471, w462) -> (→"Swerve_Overheating_Array":bool[])
            n306 = Build Array(w438, w437, w436, w435) -> (→"Swerve_Drive_Fault_Array":bool[])
            n307 = local read "Dashboard Tab"() -> (w448:T1)
            n308 = case shown="\"Tune\"" w448 {
              frame "Checklist", Default {
              }
              frame "Tune" {
                n309 = call-poly <vilib>:"NT Read Value.vi"("default value"=dbl[] [0.0, 0.0, 0.0, 0.0, 0.0, 0.0] ("Default Value"), "name"="Current_Driver_Profile_Setpoints" ("Name")) -> ("value"=w525:dbl[])  [unwired: 7 in, 2 out]
                n310 = Array To Cluster(array=w525) -> (cluster=w521:T24)
                "Current_Driver_Profile_Setpoints_GUI" <- w521
                n311 = feedback #3(dbl[] [0.0, 0.0, 0.0, 0.0, 0.0, 0.0] ("Default Value")) -> (w524:dbl[])
                n312 = feedback-in #3(w525) -> ()
                n313 = Not Equal?(x=w525, y=w524) -> (x != y?=w523:bool[])
                n314 = Or Array Elements(Boolean array=w523) -> (logical OR=w522:bool)
                n315 = case shown="True" w522 {
                  tunnel: w521 -> [_ w529]
                  frame False {
                  }
                  frame True {
                    n316 = property on="New_Driver_Profile_Setpoints_GUI" class="Clust (strict)"("Value"=w529) -> ()  [unwired: 2 in, 2 out]
                  }
                }
              }
            }
            n317 = local read "Select Driver Profile"() -> (w509:u16)
            n318 = local read "Legal_Drivers_GUI"() -> (w510:string[])
            n319 = Cluster To Array(cluster="New_Driver_Profile_Setpoints_GUI") -> (array=w452:dbl[])
            n320 = And(x="Calibrate_Wheels_GUI", y="Arm_Calibrate_Wheels_GUI") -> (x .and. y?=w455:bool)
            n321 = Not(x="Arm_Calibrate_Wheels_GUI") -> (.not. x?=w516:bool)
            n322 = To Long Integer(number=w509) -> (32bit integer=w507:i32)
            n323 = call "ReducedBWSendToNT.vim"("Value In"="Home_Wheels_GUI", "NT Name"="Home_Wheels" ("Name")) -> ()  [unwired: 1 out]
            n324 = Index Array(array=w510, index=w507) -> (element=→"Current_Driver_Profile_GUI":string)
            n325 = call "ReducedBWSendToNT.vim"("Value In"="Apply_Driver_Profile_Setpoints_GUI", "NT Name"="Apply_Driver_Profile_Setpoints" ("Name")) -> ()  [unwired: 1 out]
            n326 = call "ReducedBWSendToNT.vim"("Value In"=w452, "NT Name"="New_Driver_Profile_Setpoints" ("Name")) -> ()  [unwired: 1 out]
            n327 = call "ReducedBWSendToNT.vim"("Value In"=w455, "NT Name"="Calibrate_Wheels" ("Name")) -> ()  [unwired: 1 out]
            n328 = call "ReducedBWSendToNT.vim"("Value In"="Arm_Calibrate_Wheels_GUI", "NT Name"="Unlock_Azimuth") -> ()  [unwired: 1 out]
            n329 = Select(t=cluster{u32, u32}[] [{11776947, 16448250}, {16448250, 16448250}] ("Colors [4]"), s=w516, f=cluster{u32, u32}[] [{6618880, 16448250}, {16448250, 16448250}] ("Colors [4]")) -> (s? t:f=w515:cluster{u32, u32}[])
            n330 = property on="Calibrate_Wheels_GUI" class="Bool"("Colors [4]"=w515) -> ()  [unwired: 2 in, 2 out]
          }
          frame #7 {
            # "Arm subsystem"
            n331 = call-poly <vilib>:"NT Read Value.vi"("default value"=bool[] [FALSE, FALSE] ("Boolean array"), "name"="Elevator_Errors") -> ("value"=w575:bool[])  [unwired: 7 in, 2 out]
            n332 = Index Array(array=w575) -> (element #1=→"Elevator_Motor_Fault":bool, element #2=→"Elevator_Overheating":bool)  [unwired: 2 in]
            n333 = First Call?() -> (First Call?: T/F=w565:bool)
            n334 = call-poly <vilib>:"NT Read Value.vi"("default value"=FALSE, "name"="Elevator_Has_Arrived") -> ("value"=→"Elevator_Has_Arrived":bool)  [unwired: 7 in, 2 out]
            n335 = feedback #4() -> (w567:refnum<class "NI_Robotics_Serial Robot Arm.lvclass">)  [unwired: 1 in]
            n336 = feedback #5() -> (w566:errorcluster)  [unwired: 1 in]
            n337 = case shown="False" w565 {
              tunnel: [w634 w651] -> w568
              tunnel: [w635 w649] -> w569
              tunnel: w567 -> [w635 _]
              tunnel: w566 -> [w634 _]
              frame False {
              }
              frame True {
                n338 = expression code="(x/180.0)*pi" ("degrees to radians")(24.0 ("twist angle")) -> (w652:dbl)
                n339 = expression code="(x/180.0)*pi" ("degrees to radians")(90.0 ("twist angle")) -> (w654:dbl)
                n340 = expression code="(x/180.0)*pi" ("degrees to radians")(90.0 ("twist angle")) -> (w656:dbl)
                n341 = Bundle By Name(cluster=T15 {"twist angle"=0.0, "length"=0.0, "rotation angle"=0.0, "offset distance"=0.0, "joint type"=enum."Prismatic", "joint coordinate offset"=0.0} ("Link Parameters"), "twist angle"=w654, "rotation angle"=w656) -> (w655:T15)
                n342 = Bundle By Name(cluster=T15 {"twist angle"=0.0, "length"=0.0, "rotation angle"=0.0, "offset distance"=0.0, "joint type"=enum."Revolute", "joint coordinate offset"=0.0} ("Link Parameters"), "twist angle"=w652) -> (w653:T15)
                n343 = Build Array(w653, w655, T15 {"twist angle"=0.0, "length"=0.5, "rotation angle"=0.0, "offset distance"=0.0, "joint type"=enum."Revolute", "joint coordinate offset"=0.0} ("Link Parameters")) -> (w644:T15[])
                n344 = expression code="(x/180.0)*pi" ("degrees to radians")(cluster{"roll":dbl, "pitch":dbl, "yaw":dbl} {"roll"=0.0, "pitch"=0.0, "yaw"=0.0} ("angles")) -> (w647:cluster{"roll":dbl, "pitch":dbl, "yaw":dbl})
                n345 = call-poly <vilib>:"Initialize Serial Arm.vi"("kinematic parameters"=w644) -> ("error out"=w650:errorcluster, "serial arm out"=w648:refnum<class "NI_Robotics_Serial Robot Arm.lvclass">)  [unwired: 9 in]
                n346 = call <vilib>:"Roll Pitch Yaw to Rotation Matrix.vi"("angles"=w647) -> ("rotation matrix"=w646:T25)
                n347 = call <vilib>:"Rotation Matrix to Transform.vi"("translation vector"=dbl[] [0.0, 0.0, 0.0, 0.0] ("Default Value"), "rotation matrix"=w646) -> ("transform"=w645:T25)
                n348 = call <vilib>:"Set Base Transform.vi"("error in (no error)"=w650, "base transform"=w645, "serial arm in"=w648) -> ("error out"=w651:errorcluster, "serial arm out"=w649:refnum<class "NI_Robotics_Serial Robot Arm.lvclass">)  [unwired: 7 in]
              }
            }
            n349 = feedback-in #4(w569) -> ()
            n350 = feedback-in #5(w568) -> ()
            n351 = local read "Extender_Position (deg)"() -> (w550:dbl)
            n352 = call-poly <vilib>:"NT Read Value.vi"("default value"=0.0, "name"="Elevator_Position (in)") -> ("value"=w551:dbl)  [unwired: 7 in, 2 out]
            n353 = local read "Dashboard Tab"() -> (w564:T1)
            n354 = call-poly <vilib>:"NT Read Value.vi"("default value"=0.0, "name"="Elevator_Goal (in)") -> ("value"=w552:dbl)  [unwired: 7 in, 2 out]
            n355 = call-poly <vilib>:"NT Read Value.vi"("default value"=0.0, "name"="Wrist_Goal (deg)") -> ("value"=w553:dbl)  [unwired: 7 in, 2 out]
            n356 = Equal?(x=w564, y=T1."Tune") -> (x = y?=w562:bool)
            n357 = case shown="True" w562 {
              tunnel: w569 -> [_ w586]
              tunnel: w568 -> [_ w585]
              tunnel: w550 -> [_ w584]
              tunnel: w553 -> [_ w583]
              tunnel: w552 -> [_ w582]
              tunnel: w551 -> [_ w581]
              frame False {
              }
              frame True {
                n358 = call "Is Value Changed.vim"("value"=w584) -> ("changed or first call?"=w588:bool)
                n359 = call "Is Value Changed.vim"("value"=w583) -> ("changed or first call?"=w589:bool)
                n360 = call "Is Value Changed.vim"("value"=w582) -> ("changed or first call?"=w591:bool)
                n361 = call "Is Value Changed.vim"("value"=w581) -> ("changed or first call?"=w590:bool)
                n362 = Compound Arithmetic op=OR(w588, w589, w591, w590) -> (w580:bool)
                n363 = expression code="(x/180.0)*pi" ("degrees to radians")(w584) -> (w587:dbl)
                n364 = feedback #6() -> (w578:refnum<vi>)  [unwired: 1 in]
                n365 = case shown="True" w580 {
                  tunnel: [w592 w609] -> w579
                  tunnel: w587 -> [_ w608]
                  tunnel: w586 -> [_ w603]
                  tunnel: w585 -> [_ w602]
                  tunnel: w583 -> [_ w595]
                  tunnel: w581 -> [_ w594]
                  tunnel: w578 -> [w592 _]
                  frame False {
                  }
                  frame True {
                    w601 = 5.0  # Elevator Offset
                    w610 = 0.0  # Goal Y (in)
                    # "update the 3D arm\nsimulation graphics"
                    n366 = Sine & Cosine(0:72.3 ("x")) -> (1:w607:dbl, 2:w606:dbl)
                    n367 = Multiply(x=w595, y=w606) -> (x*y=w604:dbl)
                    n368 = Multiply(x=w595, y=w607) -> (x*y=w605:dbl)
                    n369 = expression code="(x/180.0)*pi" ("degrees to radians")(90.0 ("element")) -> (w596:dbl)
                    n370 = Add(x=w601, y=w594) -> (x+y=w600:dbl)
                    n371 = Bundle(w604, "Goal Y (in)"=w610, w605) -> (w632:cluster{dbl, "Goal Y (in)":dbl, dbl})  [unwired: 1 in]
                    n372 = expression code="x*0.0254" ("degrees to radians")(w600) -> (w599:dbl)
                    n373 = expression code="x*0.0254" ("degrees to radians")(w632) -> (w633:cluster{dbl, "Goal Y (in)":dbl, dbl})
                    n374 = Build Array(w596, w599, w608) -> (w598:dbl[])
                    n375 = call <vilib>:"Initialize Plot.vi"("error in (no error)"=w602, "serial arm in"=w603) -> ("error out"=w627:errorcluster, "serial arm out"=w628:refnum<class "NI_Robotics_Serial Robot Arm.lvclass">)  [unwired: 8 in]
                    n376 = call <vilib>:"Create Sphere.vi"("Color"=T14 {"Red"=0.0, "Green"=1.0, "Blue"=0.0, "Alpha"=1.0}, "Radius"=sgl 0.05) -> ("error out"=w631:errorcluster, "New Sphere Refnum"=w626:refnum<vi>)  [unwired: 8 in]
                    n377 = call <vilib>:"Update Plot.vi"("error in (no error)"=w627, "joint positions"=w598, "serial arm in"=w628) -> ("error out"=w629:errorcluster, "serial arm scene"=w620:refnum<vi>)  [unwired: 6 in, 1 out]
                    n378 = call <vilib>:"Create 3D Axis.vi"("Character Size"=sgl 0.1, "Axis label?"=TRUE, "Color"=T14 {"Red"=0.0, "Green"=1.0, "Blue"=1.0, "Alpha"=1.0}, "Radius"=sgl 0.01, "Length"=sgl 0.2, "Name"="XYZ axis") -> ("New Object Refnum"=w621:refnum<vi>)  [unwired: 4 in, 1 out]
                    n379 = call-poly <vilib>:"Create Object.vi"("error in (no error)"=w631, "Geometry"=w626, "Name"="goal") -> ("error out"=w624:errorcluster, "Scene:New Object"=w625:refnum<vi>)  [unwired: 7 in]
                    n380 = call-poly <vilib>:"Add Object.vi"("error in (no error)"=w629, "New Object In"=w621, "Scene Object In"=w620) -> ("error out"=w630:errorcluster, "Scene Object Out"=w622:refnum<vi>)  [unwired: 7 in]
                    n381 = call <vilib>:"Set Translation.vi"("error in (no error)"=w624, "Translation"=w633, "Scene Object"=w625) -> ("Translated Object"=w623:refnum<vi>)  [unwired: 7 in, 1 out]
                    n382 = call-poly <vilib>:"Add Object.vi"("error in (no error)"=w630, "New Object In"=w623, "Scene Object In"=w622) -> ("Scene Object Out"=w609:refnum<vi>)  [unwired: 7 in, 1 out]
                  }
                }
                n383 = feedback-in #6(w579) -> ()
              }
            }
            n384 = call "ReducedBWSendToNT.vim"("Value In"="Elevator_Override", "NT Name"="Elevator_Override") -> ()  [unwired: 1 out]
            n385 = call-poly <vilib>:"NT Read Value.vi"("name"="Wrist_Position (deg)") -> ("value"=→"Wrist_Position (deg) 2":dbl)  [unwired: 8 in, 2 out]
            n386 = call-poly <vilib>:"NT Read Value.vi"("name"="Wrist_Temp (C)") -> ("value"=→"Wrist_Temp (C) 2":dbl)  [unwired: 8 in, 2 out]
            n387 = call-poly <vilib>:"NT Read Value.vi"("name"="Extender_Position (deg)") -> ("value"=→"Extender_Position (deg)":dbl)  [unwired: 8 in, 2 out]
            n388 = call-poly <vilib>:"NT Read Value.vi"("name"="Extender_Temp (C)") -> ("value"=→"Extender_Temp (C)":dbl)  [unwired: 8 in, 2 out]
            n389 = call-poly <vilib>:"NT Read Value.vi"("name"="Pivot_Position (deg)") -> ("value"=→"Pivot_Position (deg)":dbl)  [unwired: 8 in, 2 out]
            n390 = call-poly <vilib>:"NT Read Value.vi"("name"="Pivot_Temp (C)") -> ("value"=→"Pivot_Temp (C)":dbl)  [unwired: 8 in, 2 out]
            n391 = call "ReducedBWSendToNT.vim"("Value In"="Unlock_Extender", "NT Name"="Unlock_Extender") -> ()  [unwired: 1 out]
            n392 = call "ReducedBWSendToNT.vim"("Value In"="Calibrate_Extender", "NT Name"="Calibrate_Extender") -> ()  [unwired: 1 out]
            n393 = call "ReducedBWSendToNT.vim"("Value In"="Unlock_Pivot", "NT Name"="Unlock_Pivot") -> ()  [unwired: 1 out]
            n394 = call "ReducedBWSendToNT.vim"("Value In"="Unlock_Wrist", "NT Name"="Unlock_Wrist") -> ()  [unwired: 1 out]
          }
          frame #8 {
            (unwired) FALSE ("default value")
            (unwired) FALSE ("default value")
            # "note handling subsystem"
            n395 = call-poly <vilib>:"NT Read Value.vi"("default value"=bool[] [FALSE, FALSE, FALSE, FALSE, FALSE, FALSE] ("Boolean array"), "name"="Outer_Rollers_Faults") -> ("value"=w675:bool[])  [unwired: 7 in, 2 out]
            n396 = call-poly <vilib>:"NT Read Value.vi"("default value"=bool[] [FALSE, FALSE, FALSE, FALSE, FALSE, FALSE] ("Boolean array"), "name"="Outer_Rollers_Overheating") -> ("value"=w670:bool[])  [unwired: 7 in, 2 out]
            n397 = call-poly <vilib>:"NT Read Value.vi"("default value"=bool[] [FALSE, FALSE, FALSE, FALSE, FALSE, FALSE] ("Boolean array"), "name"="Intake_Errors") -> ("value"=w677:bool[])  [unwired: 7 in, 2 out]
            n398 = Index Array(array=w675) -> (element #1=w669:bool, element #2=w657:bool)  [unwired: 2 in]
            n399 = Index Array(array=w670) -> (element #1=w659:bool, element #2=w658:bool)  [unwired: 2 in]
            n400 = Index Array(array=w677) -> (element #1=w676:bool, element #2=w668:bool)  [unwired: 2 in]
            n401 = Build Array(w668, w659, w658) -> (→"Intake_Overheating_Array":bool[])
            n402 = Build Array(w676, w669, w657) -> (→"Intake_Motor_Fault_Array":bool[])
            n403 = call-poly <vilib>:"NT Read Value.vi"("name"="Indexer_Overheating") -> ("value"=→"Indexer_Overheating":bool)  [unwired: 8 in, 2 out]
            n404 = call-poly <vilib>:"NT Read Value.vi"("name"="Indexer_Fault") -> ("value"=→"Indexer_Motor_Fault":bool)  [unwired: 8 in, 2 out]
            n405 = call-poly <vilib>:"NT Read Value.vi"("name"="Indexer_Velocity (rpm)") -> ()  [unwired: 8 in, 3 out]
            n406 = call-poly <vilib>:"NT Read Value.vi"("name"="Indexer_Temp (C)") -> ()  [unwired: 8 in, 3 out]
            n407 = call-poly <vilib>:"NT Read Value.vi"("default value"=FALSE, "name"="Intaking") -> ("value"=→"Intaking":bool)  [unwired: 7 in, 2 out]
            n408 = call-poly <vilib>:"NT Read Value.vi"("default value"=FALSE, "name"="Outtaking") -> ("value"=→"Outtaking":bool)  [unwired: 7 in, 2 out]
          }
          frame #9 {
            # "shooter subsystem"
            n409 = call-poly <vilib>:"NT Read Value.vi"("default value"=bool[] [FALSE, FALSE] ("Boolean array"), "name"="Shooter_Motor_Fault") -> ("value"=w712:bool[])  [unwired: 7 in, 2 out]
            "Shooter_Fault_Array" <- w712
            n410 = call-poly <vilib>:"NT Read Value.vi"("default value"=bool[] [FALSE, FALSE] ("Boolean array"), "name"="Shooter_Overheating") -> ("value"=w709:bool[])  [unwired: 7 in, 2 out]
            "Shooter_Overheating_Array" <- w709
            n411 = call-poly <vilib>:"NT Read Value.vi"("default value"=bool[] [FALSE, FALSE] ("Boolean array"), "name"="Wrist_Errors") -> ("value"=w701:bool[])  [unwired: 7 in, 2 out]
            n412 = Index Array(array=w701) -> (element #1=→"Wrist_Motor_Fault":bool, element #2=→"Wrist_Overheating":bool)  [unwired: 2 in]
            n413 = Index Array(array=w712) -> (element #1=→"Shooter_Motor_Left_Fault":bool, element #2=→"Shooter_Motor_Right_Fault":bool)  [unwired: 2 in]
            n414 = Index Array(array=w709) -> (element #1=→"Shooter_Left_Overheating":bool, element #2=→"Shooter_Right_Overheating":bool)  [unwired: 2 in]
            n415 = call-poly <vilib>:"NT Read Value.vi"("default value"=u16 0 ("OUT_Shooter_Selected_Targeting_State"), "name"="Shooter_States") -> ("value"=w691:i64)  [unwired: 7 in, 2 out]
            n416 = Coerce To Type(0:w691, 1:enum16{"TACO", "Subwoofer", "Stage"}."TACO" ("OUT_Shooter_Selected_Targeting_State")) -> (2:w690:enum16{"TACO", "Subwoofer", "Stage"})
            n417 = case shown="\"TACO\", Default" w690 {
              tunnel: [TRUE _ _] -> w689
              tunnel: [_ TRUE _] -> w688
              tunnel: [_ _ TRUE] -> w687
              frame "TACO", Default {
              }
              frame "Subwoofer" {
              }
              frame "Stage" {
              }
            }
            "Shooter_State_TACO" <- w689
            "Shooter_State_SUBW" <- w688
            "Shooter_State_STGE" <- w687
            n418 = call-poly <vilib>:"NT Read Value.vi"("default value"=FALSE, "name"="Ready_To_Fire") -> ("value"=→"Ready_To_Fire":bool)  [unwired: 7 in, 2 out]
            n419 = call-poly <vilib>:"NT Read Value.vi"("default value"=FALSE, "name"="Note") -> ("value"=→"Note 2":bool)  [unwired: 7 in, 2 out]
            n420 = call "ReducedBWSendToNT.vim"("Value In"="Wrist_Override", "NT Name"="Wrist_Override") -> ()  [unwired: 1 out]
          }
          frame #10 {
            w720 = FALSE ("WA_Ret_Right")
            # "combine errors for in-match reporting"
            # "manage targeting reticules"
            # "manage audible warnings"
            # "error management and driver assistance"
            n421 = local read "Swerve_Azimuth_Fault_Array"() -> (w751:bool[])
            n422 = local read "Swerve_Overheating_Array"() -> (w752:bool[])
            n423 = local read "Intake_Overheating_Array"() -> (w725:bool[])
            n424 = local read "Intake_Motor_Fault_Array"() -> (w724:bool[])
            n425 = local read "Swerve_Drive_Fault_Array"() -> (w730:bool[])
            n426 = Or Array Elements(Boolean array=w751) -> (logical OR=→"Swerve_Azimuth_Fault":bool)
            n427 = Or Array Elements(Boolean array=w752) -> (logical OR=→"Swerve_Overheating":bool)
            n428 = Or Array Elements(Boolean array=w730) -> (logical OR=→"Swerve_Drive_Fault":bool)
            n429 = Or Array Elements(Boolean array=w725) -> (logical OR=→"Intake_Overheating":bool)
            n430 = Or Array Elements(Boolean array=w724) -> (logical OR=→"Intake_Motor_Fault":bool)
            n431 = Build Array("Driver_Help", "Manipulator_Help") -> (w757:bool[])
            n432 = Or Array Elements(Boolean array=w757) -> (logical OR=w750:bool)
            n433 = Not(x=w750) -> (.not. x?=w765:bool)
            n434 = Build Array (concatenate)(w765, w757) -> (w764:bool[])
            n435 = property on="Help Graphic" class="ImageControl"("Visible"=w750) -> ()  [unwired: 2 in, 2 out]
            n436 = call "StateSelection.vi"("Disallowed States"=bool[] [FALSE, FALSE, FALSE, FALSE], "State Triggers"=w764, "State Names"=string[] ["No Help", "Driver Help", "Manipulator Help"]) -> ("Selected State"=w769:string)
            n437 = case shown="\"Driver Help\"" w769 {
              tunnel: [_ w790 w792] -> w753
              tunnel: w750 -> [_ _ _]
              frame "No Help", Default {
              }
              frame "Driver Help" {
                n438 = call "RenderJoystickDiagram.vi"("Joystick Graphic Filename"="driver joystick diagram.png") -> ("Image Out"=w790:T3)  [unwired: 10 in]
              }
              frame "Manipulator Help" {
                n439 = call "RenderJoystickDiagram.vi"("Joystick Graphic Filename"="manipulator joystick diagram.png") -> ("Image Out"=w792:T3)  [unwired: 10 in]
              }
            }
            "Help Graphic" <- w753
            n440 = Or Array Elements(Boolean array=w757) -> (logical OR=w759:bool)
            n441 = Not(x=w759) -> (.not. x?=w758:bool)
            n442 = Or(x=w758, y=w757) -> (x .or. y?=w756:bool[])
            n443 = Index Array(array=w756) -> (element #1=w732:bool, element #2=w731:bool)  [unwired: 2 in]
            n444 = Select(t=T17."Enabled" ("Disabled"), s=w731, f=T17."Disabled and Grayed Out" ("Disabled")) -> (s? t:f=w760:T17)
            n445 = Select(t=T17."Enabled" ("Disabled"), s=w732, f=T17."Disabled and Grayed Out" ("Disabled")) -> (s? t:f=w789:T17)
            n446 = property on="Driver_Help" class="Bool (strict)"("DisabledEnum"=w789) -> ()  [unwired: 2 in, 2 out]
            n447 = property on="Manipulator_Help" class="Bool (strict)"("DisabledEnum"=w760) -> ()  [unwired: 2 in, 2 out]
            n448 = First Call?() -> (First Call?: T/F=w739:bool)
            n449 = call-poly <vilib>:"NT Read Value.vi"("default value"=FALSE ("Default Value"), "name"="Master_Alarm" ("Name")) -> ("value"=w735:bool)  [unwired: 7 in, 2 out]
            n450 = call "Timer.vi"("Reset Timer"=w739) -> ("Time (ms)"=w738:u32)
            n451 = Greater?(x=w738, y=u32 2500) -> (0:w736:bool)
            n452 = local read "Arm_Calibrate_Wheels_GUI"() -> (w741:bool)
            n453 = call-poly <vilib>:"NT Read Value.vi"("default value"=0.0 ("Default Value"), "name"="Number_of_Master_Alarms" ("Name")) -> ("value"=w745:dbl)  [unwired: 7 in, 2 out]
            n454 = And(x=w736, y=w735) -> (x .and. y?=w734:bool)
            n455 = call "EdgeTrigger.vi"("Input Signal"="Mute_Audible_Warnings") -> ("Rising Edge Trigger"=w777:bool)  [unwired: 2 out]
            n456 = local read "Arm_Calibrate_Joysticks"() -> (w742:bool)
            n457 = To Long Integer(number=w745) -> (32bit integer=w744:i32)
            n458 = local read "Unlock_Extender"() -> (w721:bool)
            n459 = call "BlinkLight.vi"() -> ("Blinked"=w782:bool)  [unwired: 1 in]
            n460 = Number To Decimal String(number=w744) -> (decimal integer string=w783:string)  [unwired: 1 in]
            n461 = feedback #7(TRUE ("t")) -> (w775:bool)
            n462 = Not(x=w775) -> (.not. x?=w774:bool)
            n463 = Select(t=w774, s=w777, f=w775) -> (s? t:f=w733:bool)
            "Audible_Warnings_Enabled_GUI" <- w733
            n464 = feedback-in #7(w733) -> ()
            n465 = Select(t=w782, s=w734, f=FALSE) -> (s? t:f=w786:bool)
            "Master_Caution_GUI_1" <- w786
            "Master_Caution_GUI_0" <- w786
            "Master_Caution_GUI_2" <- w786
            n466 = Concatenate Strings("MASTER ALARM (" ("string"), w783, ")" ("string")) -> (w784:string)
            n467 = Select(t=w784, s=w786, f="") -> (s? t:f=w785:string)
            n468 = Compound Arithmetic op=OR(w742, w741, w721) -> (w740:bool)
            n469 = local read "State_Climbing"() -> (w726:bool)
            n470 = Select(t=cluster{u32, u32}[] [{6618880, 16448250}, {16448250, 16448250}] ("Colors [4]"), s=w733, f=cluster{u32, u32}[] [{16755474, 16448250}, {16448250, 16448250}] ("Colors [4]")) -> (s? t:f=w773:cluster{u32, u32}[])
            n471 = local read "State_AMP"() -> (w727:bool)
            n472 = call "ReducedBWSendToNT.vim"("Value In"=w740, "NT Name"="Some_Switch_Armed" ("Name")) -> ()  [unwired: 1 out]
            n473 = property on="Master_Caution_GUI_0" class="Bool (strict)"("BoolText.Text"=w785) -> ()  [unwired: 2 in, 2 out]
            n474 = property on="Master_Caution_GUI_1" class="Bool (strict)"("BoolText.Text"=w785) -> ()  [unwired: 2 in, 2 out]
            n475 = property on="Master_Caution_GUI_2" class="Bool (strict)"("BoolText.Text"=w785) -> ()  [unwired: 2 in, 2 out]
            n476 = property on="Mute_Audible_Warnings" class="Bool"("Colors [4]"=w773) -> ()  [unwired: 2 in, 2 out]
            n477 = Or(x=w727, y=w726) -> (x .or. y?=→"LL_Ret_Left" →"LL_Ret_Right":bool)
            "WA_Ret_Left" <- w720
            "WA_Ret_Right" <- w720
          }
          frame #11 {
            # "flush NT tables"
            n478 = call <vilib>:"NT Flush Data Updates.vi"() -> ()  [unwired: 11 in, 1 out]
          }
        }
      }
    }
  }
  n479 = while {
    stop <- FALSE stop-if-true
    # "Set window properties"
    n480 = Not(x="Dock_Dashboard") -> (.not. x?=w795:bool)
    n481 = First Call?() -> (First Call?: T/F=w799:bool)
    n482 = Wait (ms)(milliseconds to wait=u32 10) -> ()  [unwired: 1 out]
    n483 = Compound Arithmetic op=OR(w795, w799) -> (w797:bool)
    n484 = control-ref of="This VI"() -> (w798:refnum<vi>)
    n485 = call "EdgeTrigger.vi"("Input Signal"=w797) -> ("Falling Edge Trigger"=w796:bool)  [unwired: 2 out]
    n486 = case shown="False" w797 {
      tunnel: w798 -> [w804 w811]
      tunnel: w796 -> [w802 _]
      frame False {
        n487 = case shown="True" w802 {
          tunnel: T26 {"Left"=100, "Top"=100, "Right"=1390, "Bottom"=585} ("Front Panel Window:Window Bounds") -> [_ w810]
          tunnel: w804 -> [w807 w809]
          tunnel: [w807 w808] -> w803
          frame False {
          }
          frame True {
            n488 = property class="VI"(reference=w809, "Front Panel.WinBounds"=w810) -> (reference out=w808:refnum<vi>)  [unwired: 1 in, 1 out]
          }
        }
        n489 = property class="VI"(reference=w803, "Front Panel.TitleBarVis"=TRUE ("Front Panel Window:Title Bar Visible")) -> ()  [unwired: 1 in, 2 out]
      }
      frame True {
        n490 = property class="VI"(reference=w811, "Front Panel.WinBounds"=T26 {"Left"=0, "Top"=0, "Right"=1290, "Bottom"=485} ("Front Panel Window:Window Bounds"), "Front Panel.TitleBarVis"=FALSE ("Front Panel Window:Title Bar Visible")) -> ()  [unwired: 1 in, 2 out]
      }
    }
  }
  n491 = while {
    tunnel: w20 -> [w817]
    tunnel: w19 -> [_]
    tunnel: w17 -> [w816]
    tunnel: w12 -> [w815]
    tunnel: w5 -> [w814]
    stop <- FALSE stop-if-true
    # "Process UI events related to test mode, checklist, and camera settings"
    n492 = event shown="[0] Timeout" {
      selector: w817 -> [_ _ _ _]
      dyn-events: _ -> [_ _ _ _]
      timeout: u32 60 ("milliseconds to wait") -> [_ _ _ _]
      tunnel: w816 -> [_ _ _ _]
      tunnel: w815 -> [_ _ _ _]
      tunnel: w814 -> [w820 _ _ _]
      event Timeout {
        (unwired) T1."Variables" ("Dashboard Tab")
        n493 = event-data() -> ()  [unwired: 1 in, 1 out]
        n494 = case shown="\"Variables\"" "Dashboard Tab" {
          tunnel: w820 -> [_ _ _]
          frame "Tune" {
          }
          frame "TeleOp", Default {
          }
          frame "Variables" {
            w825 = string[] ["CameraPublisher", "Usage", "DB"]  # Items to initially close
            n495 = First Call?() -> (First Call?: T/F=w826:bool)
            n496 = control-ref of="Tree"() -> (w827:refnum<vi>)
            n497 = Select(t=w825, s=w826, f=string[] []) -> (s? t:f=w823:string[])
            n498 = call <vilib>:"NT Read and Format Entries as Tree.vi"("Tags to  Close"=w823, "Tree Refnum"=w827) -> ()  [unwired: 8 in, 2 out]
          }
        }
        n499 = call <vilib>:"Connextion Info.vi"() -> ("Connected"=→"NT Connection":bool)  [unwired: 10 in, 1 out]
      }
      event "CheckList": Double Click {
        # "Shift clears all"
        # "Update symbols on the listbox"
        n500 = event-data() -> ("PlatMods.Shift"=w828:bool, "Row"=w830:i32)  [unwired: 1 in]
        n501 = case shown="False" w828 {
          tunnel: w830 -> [w834 _]
          tunnel: 1 -> [w833 _]
          frame False {
            n502 = property on="CheckList" class="LstBox (strict)"() -> ("Item Symbols"=w832:i32[])  [unwired: 2 in, 2 out]
            n503 = Replace Array Subset(array=w832, new element=w833, index=w834) -> (w831:i32[])
            n504 = property on="CheckList" class="LstBox (strict)"("Item Symbols"=w831) -> ()  [unwired: 2 in, 2 out]
          }
          frame True {
            w835 = 0 ("Top Row")
            n505 = property on="CheckList" class="LstBox (strict)"() -> ("Number of Rows"=w837:u32)  [unwired: 2 in, 2 out]
            n506 = Initialize Array(0, w837) -> (w836:i32[])
            n507 = property on="CheckList" class="LstBox (strict)"("Top Row"=w835, "Value"=w835, "Item Symbols"=w836) -> ()  [unwired: 2 in, 2 out]
          }
        }
      }
      event "CheckList": Key Down {
        # "Update symbols on the listbox\nLeft and right keys check and uncheck"
        n508 = event-data() -> ("VKey"=w840:T27)  [unwired: 1 in]
        n509 = case shown="\"Left\", \"Right\"" w840 {
          selector: w840 -> [w845 _]
          tunnel: eventvkey."Left" ("VKey") -> [w843 _]
          frame "Left", "Right" {
            n510 = Equal?(x=w843, y=w845) -> (x = y?=w844:bool)
            n511 = Select(t=0, s=w844, f=1) -> (s? t:f=w846:i32)
            n512 = property on="CheckList" class="LstBox (strict)"() -> ("Item Symbols"=w849:i32[])  [unwired: 2 in, 2 out]
            n513 = Replace Array Subset(array=w849, new element=w846, index="CheckList") -> (w848:i32[])
            n514 = property on="CheckList" class="LstBox (strict)"("Item Symbols"=w848) -> ()  [unwired: 2 in, 2 out]
          }
          frame Default {
          }
        }
      }
      event "Tree": Double Click {
        n515 = event-data() -> ("PlatMods"=w855:T28, "Tag"=w852:string)  [unwired: 1 in]
        n516 = Unbundle(w855) -> ("Shift"=w854:bool)  [unwired: 4 out]
        n517 = String Subset(string=w852, length (rest)=1 ("length (rest)")) -> (substring=w851:string)  [unwired: 1 in]
        n518 = Not(x=w854) -> (.not. x?=w853:bool)
        n519 = case shown="\"/\"" w851 {
          tunnel: w852 -> [_ w857]
          tunnel: w853 -> [_ w856]
          frame Default {
          }
          frame "/" {
            n520 = call <vilib>:"NT Update Persistence.vi"("Persistence"=w856, "Name"=w857) -> ()  [unwired: 9 in, 1 out]
          }
        }
      }
    }
  }
  n521 = while {
    tunnel: u16 1741 ("timeout ms (25000)") -> [w859]
    stop <- FALSE stop-if-true
    # "Wait for DS connections"
    n522 = TCP Create Listener(10:w859) -> (0:w858:errorcluster, 3:w860:refnum<k5>)  [unwired: 4 in, 1 out]
    n523 = case shown="No Error" w858 {
      selector: w858 -> [w862 _]
      tunnel: w860 -> [w863 _]
      frame No Error {
        n524 = while {
          tunnel: w863 -> [w866]
          tunnel: w862 -> [w865]
          stop <- FALSE stop-if-true
          n525 = TCP Wait On Listener(8:w865, 11:w866) -> (0:w867:errorcluster, 4:w868:refnum<k5>)  [unwired: 2 in, 3 out]
          n526 = local write "TCP"(w868) -> ()
          n527 = case shown="Error" w867 {
            frame No Error {
            }
            frame Error {
              n528 = Wait (ms)(milliseconds to wait=u32 1000) -> ()  [unwired: 1 out]
            }
          }
        }
      }
      frame Error {
        n529 = Wait (ms)(milliseconds to wait=u32 1000) -> ()  [unwired: 1 out]
      }
    }
  }
  n530 = while {
    shift-right: [w882] -> _
    shift-left: _ -> [w934]
    shift-right: [w883] -> _
    shift-left: _ -> [w924]
    tunnel: w4 -> [_]
    stop <- FALSE stop-if-true
    # "Dynamic Overlays"
    n531 = To Long Integer(number="Reticule") -> (32bit integer=w915:i32)
    n532 = Wait (ms)(milliseconds to wait=u32 100) -> ()  [unwired: 1 out]
    n533 = Multiply(x=w915, y=2) -> (x*y=w914:i32)
    n534 = control-ref of="WA_Ret_Left"() -> (w896:refnum<vi>)
    n535 = control-ref of="WA_Ret_Right"() -> (w895:refnum<vi>)
    n536 = control-ref of="LL_Ret_Left"() -> (w881:refnum<vi>)
    n537 = control-ref of="LL_Ret_Right"() -> (w880:refnum<vi>)
    n538 = Increment(x=w914) -> (x+1=w902:i32)
    n539 = First Call?() -> (First Call?: T/F=w905:bool)
    n540 = Index Array(array=w924, index #1=w914, index #2=w902) -> (element #1=w918:i32, element #2=w926:i32)
    n541 = Or(x="Up", y="Down") -> (x .or. y?=w930:bool)
    n542 = Or(x="Left", y="Right") -> (x .or. y?=w920:bool)
    n543 = case shown="True" w905 {
      tunnel: [w945 w958] -> w882
      tunnel: w934 -> [w945 _]
      tunnel: w896 -> [_ w957]
      tunnel: w895 -> [_ w956]
      tunnel: w881 -> [_ w947]
      tunnel: w880 -> [_ w946]
      frame False {
      }
      frame True {
        n544 = property class="Bool (strict)"(reference=w957) -> ("Left"=w955:i32, "Top"=w954:i32)  [unwired: 1 in, 2 out]
        n545 = property class="Bool (strict)"(reference=w956) -> ("Left"=w953:i32, "Top"=w952:i32)  [unwired: 1 in, 2 out]
        n546 = property class="Bool (strict)"(reference=w947) -> ("Left"=w951:i32, "Top"=w950:i32)  [unwired: 1 in, 2 out]
        n547 = property class="Bool (strict)"(reference=w946) -> ("Left"=w949:i32, "Top"=w948:i32)  [unwired: 1 in, 2 out]
        n548 = Build Array(w955, w954, w953, w952, w951, w950, w949, w948) -> (w958:i32[])
      }
    }
    n549 = Bundle("WA_Ret_Left"=w896, "WA_Ret_Right"=w895, "LL_Ret_Left"=w881, "LL_Ret_Right"=w880) -> (w887:T29)  [unwired: 1 in]
    n550 = Decrement(x=w926) -> (x-1=w933:i32)
    n551 = Increment(x=w926) -> (x+1=w932:i32)
    n552 = Decrement(x=w918) -> (x-1=w923:i32)
    n553 = Increment(x=w918) -> (x+1=w922:i32)
    n554 = Select(t=w933, s="Up", f=w932) -> (s? t:f=w931:i32)
    n555 = Select(t=w923, s="Left", f=w922) -> (s? t:f=w921:i32)
    n556 = Select(t=w931, s=w930, f=w926) -> (s? t:f=w901:i32)
    n557 = Select(t=w921, s=w920, f=w918) -> (s? t:f=w919:i32)
    n558 = Replace Array Subset(array=w924, new element #1=w919, index #1=w914, new element #2=w901, index #2=w902) -> (w900:i32[])
    n559 = Current VI's Path() -> (path=w910:path)
    n560 = Strip Path(path=w910) -> (stripped path=w909:path)  [unwired: 1 out]
    n561 = Cluster To Array(cluster=w887) -> (array=w899:refnum<vi>[])
    n562 = Strip Path(path=w909) -> (stripped path=w871:path)  [unwired: 1 out]
    n563 = Array Size(array=w899) -> (size(s)=w898:i32)
    n564 = Build Path(base path=w871, name or relative path=path "reticule positions" ("XML File Path")) -> (appended path=w908:path)
    n565 = Multiply(x=2 ("dimension size"), y=w898) -> (x*y=w904:i32)
    n566 = Initialize Array(0, w904) -> (w894:i32[])
    n567 = call-poly <vilib>:"Read From XML File.vi"("XML File Path"=w908) -> ("error out"=w886:errorcluster, "XML Elements"=w907:string[])  [unwired: 8 in, 1 out]
    n568 = case shown="No Error" w886 {
      tunnel: w907 -> [w941 _]
      tunnel: w894 -> [w938 _]
      tunnel: [w937 i32[] [0, 0, 0, 0, 0, 0, 0, 0, 0, 0, 0, 0] ("value")] -> w884
      frame No Error {
        n569 = Index Array(array=w941, index=0) -> (element=w939:string)
        n570 = Unflatten From XML(xml string=w939, type=w938) -> (value=w937:i32[])  [unwired: 1 in, 1 out]
      }
      frame Error {
      }
    }
    n571 = First Call?() -> (First Call?: T/F=w925:bool)
    n572 = Select(t=w884, s=w925, f=w900) -> (s? t:f=w883:i32[])
    n573 = Add(x=w883, y=w882) -> (x+y=w885:i32[])
    n574 = Index Array(array=w885, index #1=0 ("index")) -> (element #1=w891:i32, element #2=w890:i32, element #3=w889:i32, element #4=w888:i32, element #5=w879:i32, element #6=w878:i32, element #7=w877:i32, element #8=w876:i32)  [unwired: 7 in]
    n575 = Unbundle(w887) -> ("WA_Ret_Left"=w892:refnum<vi>, "WA_Ret_Right"=w893:refnum<vi>, "LL_Ret_Left"=w875:refnum<vi>, "LL_Ret_Right"=w874:refnum<vi>)
    n576 = Flatten To XML(6:w883) -> (2:w912:string)
    n577 = call "EdgeTrigger.vi"("Input Signal"="Save") -> ("Rising Edge Trigger"=w872:bool)  [unwired: 2 out]
    n578 = case shown="True" w872 {
      tunnel: w912 -> [_ w944]
      tunnel: w908 -> [_ w943]
      frame False {
      }
      frame True {
        n579 = call-poly <vilib>:"Write to XML File.vi"("XML Input"=w944, "XML File Path"=w943) -> ()  [unwired: 7 in, 3 out]
      }
    }
    n580 = property class="Bool (strict)"(reference=w892, "Left"=w891, "Top"=w890) -> ()  [unwired: 1 in, 2 out]
    n581 = property class="Bool (strict)"(reference=w893, "Left"=w889, "Top"=w888) -> ()  [unwired: 1 in, 2 out]
    n582 = property class="Bool (strict)"(reference=w875, "Left"=w879, "Top"=w878) -> ()  [unwired: 1 in, 2 out]
    n583 = property class="Bool (strict)"(reference=w874, "Left"=w877, "Top"=w876) -> ()  [unwired: 1 in, 2 out]
  }
  n584 = while {
    stop <- FALSE stop-if-true
    # "Error Message Handling"
    n585 = property on="Actuator Testing" class="Ring (strict)"() -> ("RingText.Text"=w1036:string)  [unwired: 2 in, 2 out]
    n586 = local read "(Back) Lime_Vision_Fault_GUI"() -> (w1008:bool)
    n587 = local read "Intake_Overheating_Array"() -> (w978:bool[])
    n588 = local read "Intake_Motor_Fault_Array"() -> (w986:bool[])
    n589 = local read "Shooter_Overheating_Array"() -> (w976:bool[])
    n590 = local read "Shooter_Fault_Array"() -> (w970:bool[])
    n591 = local read "Master_Safety_Override_1"() -> (w1011:bool)
    n592 = local read "Wrist_Overheating"() -> (w961:bool)
    n593 = local read "Wrist_Motor_Fault"() -> (w965:bool)
    n594 = local read "Arm_Calibrate_Wheels_GUI"() -> (w1056:bool)
    n595 = local read "Arm_Calibrate_Joysticks"() -> (w1026:bool)
    n596 = local read "CAN_Bus_Fault_GUI"() -> (w1023:bool)
    n597 = Wait (ms)(milliseconds to wait=u32 200) -> ()  [unwired: 1 out]
    n598 = local read "Elevator_Overheating"() -> (w988:bool)
    n599 = local read "Elevator_Motor_Fault"() -> (w994:bool)
    n600 = local read "Swerve_Azimuth_Fault"() -> (w1060:bool)
    n601 = Not Equal?(x=w1036, y="No_Test") -> (x != y?=w1043:bool)
    n602 = local read "Home_Wheels_GUI"() -> (w1013:bool)
    n603 = local read "Swerve_Overheating"() -> (w1069:bool)
    n604 = local read "Super_Test_Mode_GUI"() -> (w1077:bool)
    n605 = call <vilib>:"Space Constant.vi"() -> ("String"=w1034:string)
    n606 = local read "Swerve_Drive_Fault"() -> (w1004:bool)
    n607 = local read "Auto_Test_Mode_GUI"() -> (w1048:bool)
    n608 = local read "Elevator_Override"() -> (w996:bool)
    n609 = local read "Wrist_Override"() -> (w1002:bool)
    n610 = local read "IMU_Failure_GUI"() -> (w1040:bool)
    n611 = local read "Electrical_Fault_GUI"() -> (w1031:bool)
    n612 = local read "Pressure_Vent_GUI"() -> (w1065:bool)
    n613 = local read "Auto_Error_GUI"() -> (w1053:bool)
    n614 = Search and Replace String(replace all?=TRUE ("replace all? (F)"), input string=w1036, search string="_", replace string=w1034) -> (result string=w1037:string)  [unwired: 4 in, 3 out]
    n615 = local read "Slow_Loop"() -> (w1072:bool)
    n616 = Or Array Elements(Boolean array=w986) -> (logical OR=w983:bool)
    n617 = Or Array Elements(Boolean array=w978) -> (logical OR=w981:bool)
    n618 = Or Array Elements(Boolean array=w976) -> (logical OR=w973:bool)
    n619 = Or Array Elements(Boolean array=w970) -> (logical OR=w972:bool)
    n620 = Concatenate Strings("testing " ("string"), w1037) -> (w1046:string)
    n621 = Bundle("homing the wheels", "Home_Wheels_GUI"=w1013, 60.0) -> (w1012:cluster{string, "Home_Wheels_GUI":bool, dbl})  [unwired: 1 in]
    n622 = Bundle("Lime Light failure", "(Back) Lime_Vision_Fault_GUI"=w1008, 600.0) -> (w1007:T30)  [unwired: 1 in]
    n623 = Bundle("swerve drive failure", "Swerve_Drive_Fault"=w1004, 600.0) -> (w1003:cluster{string, "Swerve_Drive_Fault":bool, dbl})  [unwired: 1 in]
    n624 = Bundle("Wrist Override", "Wrist_Override"=w1002, 600.0) -> (w999:cluster{string, "Wrist_Override":bool, dbl})  [unwired: 1 in]
    n625 = Bundle("Elevator Override", "Elevator_Override"=w996, 600.0) -> (w995:cluster{string, "Elevator_Override":bool, dbl})  [unwired: 1 in]
    n626 = Bundle("Elevator Motor Failure", "Elevator_Motor_Fault"=w994, 600.0) -> (w991:T31)  [unwired: 1 in]
    n627 = Bundle("Elevator Overheating", "Elevator_Overheating"=w988, 600.0) -> (w987:T32)  [unwired: 1 in]
    n628 = Bundle("Intake Motor Fault", w983, 600.0) -> (w982:cluster{string, bool, dbl})  [unwired: 1 in]
    n629 = Bundle("Intake Overheating", w981, 600.0) -> (w977:cluster{string, bool, dbl})  [unwired: 1 in]
    n630 = Bundle("Shooter Overheating", w973, 600.0) -> (w968:cluster{string, bool, dbl})  [unwired: 1 in]
    n631 = Bundle("Shooter Motor Fault", w972, 600.0) -> (w967:cluster{string, bool, dbl})  [unwired: 1 in]
    n632 = Bundle("Wrist Motor Fault", "Wrist_Motor_Fault"=w965, 600.0) -> (w963:cluster{string, "Wrist_Motor_Fault":bool, dbl})  [unwired: 1 in]
    n633 = Bundle("Wrist Overheating", "Wrist_Overheating"=w961, 600.0) -> (w959:cluster{string, "Wrist_Overheating":bool, dbl})  [unwired: 1 in]
    n634 = Bundle("safeties disengaged", "Master_Safety_Override_1"=w1011, 10.0) -> (w1081:T33)  [unwired: 1 in]
    n635 = Bundle("disabled test mode", "Super_Test_Mode_GUI"=w1077, 10.0) -> (w1080:cluster{string, "Super_Test_Mode_GUI":bool, dbl})  [unwired: 1 in]
    n636 = Bundle("control latency too high", "Slow_Loop"=w1072, 60.0) -> (w1073:cluster{string, "Slow_Loop":bool, dbl})  [unwired: 1 in]
    n637 = Bundle("drive train overheating", "Swerve_Overheating"=w1069, 60.0) -> (w1068:cluster{string, "Swerve_Overheating":bool, dbl})  [unwired: 1 in]
    n638 = Bundle("pressure venting", "Pressure_Vent_GUI"=w1065, 600.0) -> (w1064:cluster{string, "Pressure_Vent_GUI":bool, dbl})  [unwired: 1 in]
    n639 = Bundle("swerve azimuth failure", "Swerve_Azimuth_Fault"=w1060, 600.0) -> (w1061:T34)  [unwired: 1 in]
    n640 = Bundle("ready to calibrate swerve modules", "Arm_Calibrate_Wheels_GUI"=w1056, 10.0) -> (w1057:T35)  [unwired: 1 in]
    n641 = Bundle("autonomous play failure", "Auto_Error_GUI"=w1053, 10.0) -> (w1052:cluster{string, "Auto_Error_GUI":bool, dbl})  [unwired: 1 in]
    n642 = Bundle("autonomous test mode", "Auto_Test_Mode_GUI"=w1048, 10.0) -> (w1049:cluster{string, "Auto_Test_Mode_GUI":bool, dbl})  [unwired: 1 in]
    n643 = Bundle(w1046, w1043, 10.0) -> (w1042:cluster{string, bool, dbl})  [unwired: 1 in]
    n644 = Bundle("IMU failure, auto-targeting disabled", "IMU_Failure_GUI"=w1040, 600.0) -> (w1038:cluster{string, "IMU_Failure_GUI":bool, dbl})  [unwired: 1 in]
    n645 = Bundle("electrical bus fault, power down", "Electrical_Fault_GUI"=w1031, 60.0) -> (w1030:T36)  [unwired: 1 in]
    n646 = Bundle("ready to calibrate joysticks, wait ten seconds after pressing calibrate", "Arm_Calibrate_Joysticks"=w1026, 10.0) -> (w1027:T37)  [unwired: 1 in]
    n647 = Bundle("CAN bus fault, check wiring", "CAN_Bus_Fault_GUI"=w1023, 60.0) -> (w1025:cluster{string, "CAN_Bus_Fault_GUI":bool, dbl})  [unwired: 1 in]
    n648 = local read "Audible_Warnings_Enabled_GUI"() -> (w1019:bool)
    n649 = Build Array(w1081, w1080, w1073, w1068, w1064, w1061, w1057, w1052, w1049, w1042, w1038, w1030, w1027, w1025, w1012, w1007, w1003, w999, w995, w991, w987, w982, w977, w968, w967, w963, w959) -> (w1079:cluster{string, "Wrist_Overheating":bool, dbl}[])
    n650 = call "EdgeTrigger.vi"("Input Signal"=w1019) -> ("All Edge Trigger"=w1018:bool)  [unwired: 2 out]
    n651 = call "ErrorMessageBuilder.vi"("Errors"=w1079, "Reset Error History"=w1018) -> ("Combined Error String"=w1020:string)
    n652 = Not Equal?(x="", y=w1020) -> (x != y?=w1021:bool)
    n653 = Compound Arithmetic op=AND(w1019, w1021) -> (w1017:bool)
    n654 = case shown="True" w1017 {
      tunnel: w1020 -> [_ w1088]
      frame False {
      }
      frame True {
        n655 = call "TextToSpeech.vi"("Text To Be Spoken"=w1088) -> ()  [unwired: 9 in, 2 out]
      }
    }
    n656 = case shown="True" w1021 {
      tunnel: w1020 -> [_ w1087]
      frame False {
      }
      frame True {
        "Combined Error String" <- w1087
      }
    }
  }
